vi "IcRn Curve Array.vi"() -> ()   [LabVIEW 2016]
panel:
  out "SC-fitting Clusters":cluster{"Rn":dbl, "Rc":dbl, "Rn/Rc ratio":dbl}[](array[cluster])=[{"Rn"=26609.67786588797, "Rc"=2146.640191844906, "Rn/Rc ratio"=12.39596554978251}, {"Rn"=26578.792114511656, "Rc"=2137.411881992016, "Rn/Rc ratio"=12.435035258501918}, {"Rn"=26563.358623435608, "Rc"=2083.2272039529967, "Rn/Rc ratio"=12.751061705142245}, {"Rn"=25938.706790932443, "Rc"=2244.184409808236, "Rn/Rc ratio"=11.558188657566197}, {"Rn"=25908.041740086435, "Rc"=2057.919835889771, "Rn/Rc ratio"=12.589431953691589}, {"Rn"=25865.50185276808, "Rc"=2204.392899899708, "Rn/Rc ratio"=11.733616930967646}, {"Rn"=25488.748575504553, "Rc"=2145.43014835337, "Rn/Rc ratio"=11.880484011594278}, {"Rn"=25365.459659139524, "Rc"=2113.116572134784, "Rn/Rc ratio"=12.003814646872025}, {"Rn"=25357.80891823078, "Rc"=2012.1993643655096, "Rn/Rc ratio"=12.602036044388997}, {"Rn"=24803.296836656464, "Rc"=1935.449110044589, "Rn/Rc ratio"=12.815266858700845}, {"Rn"=24789.427309484585, "Rc"=2110.7215877648796, "Rn/Rc ratio"=11.744527299659174}, {"Rn"=24753.340817673175, "Rc"=1907.8722974852653, "Rn/Rc ratio"=12.974317437440725}, {"Rn"=24193.381040172608, "Rc"=1986.2611655574085, "Rn/Rc ratio"=12.18036251208847}, {"Rn"=24141.67211311363, "Rc"=1914.2262988636805, "Rn/Rc ratio"=12.611712694285186}, {"Rn"=24054.376770789982, "Rc"=2034.7991063607624, "Rn/Rc ratio"=11.821499574870185}, {"Rn"=23498.377622554053, "Rc"=1747.9097873838214, "Rn/Rc ratio"=13.443701609866936}, {"Rn"=23433.481724089263, "Rc"=1853.1661496580136, "Rn/Rc ratio"=12.645105636326088}, {"Rn"=23378.696455272377, "Rc"=1802.771292074766, "Rn/Rc ratio"=12.968198771551547}, {"Rn"=22737.05296381861, "Rc"=1678.3245594247633, "Rn/Rc ratio"=13.547470801244552}, {"Rn"=22680.76965817146, "Rc"=1749.9212441766977, "Rn/Rc ratio"=12.961023093837746}, {"Rn"=22666.430402112397, "Rc"=1723.1362618386952, "Rn/Rc ratio"=13.154171787857267}, {"Rn"=22027.13711147753, "Rc"=1754.0754738398637, "Rn/Rc ratio"=12.557690612512646}, {"Rn"=21965.31458464643, "Rc"=1772.3528948958199, "Rn/Rc ratio"=12.393307590099072}, {"Rn"=21904.088799010322, "Rc"=1647.9899361875666, "Rn/Rc ratio"=13.2913971851569}, {"Rn"=21327.67605888909, "Rc"=1699.7562893724967, "Rn/Rc ratio"=12.547490597468348}, {"Rn"=21242.85250961181, "Rc"=1778.1623981981945, "Rn/Rc ratio"=11.946519919180112}, {"Rn"=21190.69234118089, "Rc"=1678.9409582743576, "Rn/Rc ratio"=12.621463689206214}, {"Rn"=20522.79001382321, "Rc"=1750.8462305265753, "Rn/Rc ratio"=11.721640459339987}, {"Rn"=20484.445522882474, "Rc"=1809.3684443337136, "Rn/Rc ratio"=11.321323518729606}, {"Rn"=20413.32456904895, "Rc"=1657.0773651102954, "Rn/Rc ratio"=12.318872370627206}, {"Rn"=19783.027782642876, "Rc"=1735.823288979653, "Rn/Rc ratio"=11.396913446340314}, {"Rn"=19715.891712150584, "Rc"=1800.9327427343387, "Rn/Rc ratio"=10.947600231986529}, {"Rn"=19681.22954295286, "Rc"=1875.9645987166225, "Rn/Rc ratio"=10.491258500516004}, {"Rn"=19073.25011455856, "Rc"=1794.1581209072158, "Rn/Rc ratio"=10.630752045931255}, {"Rn"=18990.747145177967, "Rc"=1751.6053469823771, "Rn/Rc ratio"=10.841909781729521}, {"Rn"=18936.08683536125, "Rc"=1762.5785362990346, "Rn/Rc ratio"=10.743400333878002}, {"Rn"=18450.3221338972, "Rc"=1708.93301365366, "Rn/Rc ratio"=10.796398680631038}, {"Rn"=18428.466285582617, "Rc"=1674.3218759950107, "Rn/Rc ratio"=11.006525417719342}, {"Rn"=18355.767337683894, "Rc"=1858.6237983654753, "Rn/Rc ratio"=9.875999303262155}, {"Rn"=17859.23397265431, "Rc"=1739.1190161552418, "Rn/Rc ratio"=10.269126958393349}, {"Rn"=17778.957863612708, "Rc"=1743.0073597486146, "Rn/Rc ratio"=10.200162244970027}, {"Rn"=17766.767929712023, "Rc"=1826.0747012887841, "Rn/Rc ratio"=9.729485829453097}, {"Rn"=17124.26563957245, "Rc"=1800.6179257907434, "Rn/Rc ratio"=9.51021612875053}, {"Rn"=17040.07209132531, "Rc"=1840.0009129073826, "Rn/Rc ratio"=9.260904150531273}, {"Rn"=16996.11181161611, "Rc"=1842.768006105162, "Rn/Rc ratio"=9.22314244403383}, {"Rn"=16503.730435302114, "Rc"=1885.2441857597194, "Rn/Rc ratio"=8.754160633388405}, {"Rn"=16378.924486528076, "Rc"=1866.7278065970531, "Rn/Rc ratio"=8.77413644809095}, {"Rn"=16336.813010769789, "Rc"=1877.4399266184203, "Rn/Rc ratio"=8.701643540837598}, {"Rn"=15797.875553425325, "Rc"=1812.5608870279023, "Rn/Rc ratio"=8.7157764831445}, {"Rn"=15734.825878147443, "Rc"=1872.8361883043326, "Rn/Rc ratio"=8.401602861163083}, {"Rn"=15694.731752981366, "Rc"=1910.4003923466507, "Rn/Rc ratio"=8.215414850131316}, {"Rn"=15300.779487653343, "Rc"=1885.4328596855091, "Rn/Rc ratio"=8.115260858562483}, {"Rn"=15231.177407861678, "Rc"=1936.904865101264, "Rn/Rc ratio"=7.863668310351098}, {"Rn"=15191.108179437479, "Rc"=1919.9426274461057, "Rn/Rc ratio"=7.912271940982208}, {"Rn"=14806.152885467243, "Rc"=1867.241081445293, "Rn/Rc ratio"=7.929427556299745}, {"Rn"=14756.205731190325, "Rc"=1834.3880543575835, "Rn/Rc ratio"=8.044211635666183}, {"Rn"=14732.965553995622, "Rc"=1901.6404450592686, "Rn/Rc ratio"=7.747503263444966}, {"Rn"=14331.684473181096, "Rc"=1980.624550270427, "Rn/Rc ratio"=7.23594205233107}, {"Rn"=14240.534552208328, "Rc"=1957.7503878737575, "Rn/Rc ratio"=7.273927585668601}, {"Rn"=14224.099719417836, "Rc"=1933.6717752448858, "Rn/Rc ratio"=7.356005244280124}, {"Rn"=13925.05115218171, "Rc"=1968.8315523994395, "Rn/Rc ratio"=7.072748877480695}, {"Rn"=13914.525766155477, "Rc"=1952.9090448194245, "Rn/Rc ratio"=7.125024999534519}, {"Rn"=13900.160543802975, "Rc"=1970.0644207332862, "Rn/Rc ratio"=7.055688330551717}, {"Rn"=13569.240810667905, "Rc"=2016.888834974567, "Rn/Rc ratio"=6.727807985926509}, {"Rn"=13555.992121061312, "Rc"=1964.544925126344, "Rn/Rc ratio"=6.900321773089256}, {"Rn"=13556.977493365734, "Rc"=2007.8894139072875, "Rn/Rc ratio"=6.751854658660855}, {"Rn"=13267.959781743146, "Rc"=2017.4672930967038, "Rn/Rc ratio"=6.576542691493918}, {"Rn"=13233.202853717605, "Rc"=2004.1695247062132, "Rn/Rc ratio"=6.60283608276971}, {"Rn"=13204.171960570418, "Rc"=2007.485522874923, "Rn/Rc ratio"=6.57746808637539}, {"Rn"=12929.525312561722, "Rc"=2011.982125208965, "Rn/Rc ratio"=6.426262515239223}, {"Rn"=12902.37901238455, "Rc"=2032.3267630250373, "Rn/Rc ratio"=6.348575065350158}, {"Rn"=12867.464844428734, "Rc"=2084.56046668184, "Rn/Rc ratio"=6.172747229017011}, {"Rn"=12635.505659805094, "Rc"=2052.0589191286263, "Rn/Rc ratio"=6.157477030518479}, {"Rn"=12578.747677887168, "Rc"=2023.2906359397762, "Rn/Rc ratio"=6.216975186090654}, {"Rn"=12564.870248569116, "Rc"=2027.8736517600116, "Rn/Rc ratio"=6.196081416445221}, {"Rn"=12287.456007341623, "Rc"=2093.781580679471, "Rn/Rc ratio"=5.868547187884858}, {"Rn"=12260.101827231643, "Rc"=2057.114850581173, "Rn/Rc ratio"=5.95985286080062}, {"Rn"=12239.950999851239, "Rc"=2059.2985694862946, "Rn/Rc ratio"=5.943747633887093}, {"Rn"=11968.212813789605, "Rc"=2113.6196057668526, "Rn/Rc ratio"=5.662425150266034}, {"Rn"=11901.353165405668, "Rc"=2068.2746198260493, "Rn/Rc ratio"=5.754242232304056}, {"Rn"=11872.797453714444, "Rc"=2091.1697936758906, "Rn/Rc ratio"=5.6775865305725635}, {"Rn"=11654.569767254134, "Rc"=2073.6782578342772, "Rn/Rc ratio"=5.6202401328285205}, {"Rn"=11583.170493913314, "Rc"=2137.4139727042425, "Rn/Rc ratio"=5.419245238328053}, {"Rn"=11565.794206204415, "Rc"=2090.415090416247, "Rn/Rc ratio"=5.532773973565898}, {"Rn"=11389.764008623597, "Rc"=2169.6812982806573, "Rn/Rc ratio"=5.24951015508559}, {"Rn"=11336.004809315062, "Rc"=2221.1633517014097, "Rn/Rc ratio"=5.103634003609725}, {"Rn"=11312.595295934347, "Rc"=2232.5217076006597, "Rn/Rc ratio"=5.067182664974954}, {"Rn"=11107.690306718008, "Rc"=2265.135879507835, "Rn/Rc ratio"=4.903763349124764}, {"Rn"=11098.45825051801, "Rc"=2293.6519573759015, "Rn/Rc ratio"=4.838771730308823}, {"Rn"=11042.554973244516, "Rc"=2261.662027967936, "Rn/Rc ratio"=4.882495632278913}, {"Rn"=10869.313335071296, "Rc"=2236.1809824862203, "Rn/Rc ratio"=4.860659052285932}, {"Rn"=10827.650137466882, "Rc"=2257.009387478776, "Rn/Rc ratio"=4.797343864644738}, {"Rn"=10767.742631637293, "Rc"=2256.68945035892, "Rn/Rc ratio"=4.771477364740955}, {"Rn"=10550.21488969895, "Rc"=2365.489605338067, "Rn/Rc ratio"=4.460055485296098}, {"Rn"=10477.3548184157, "Rc"=2334.973260367238, "Rn/Rc ratio"=4.487141243222569}, {"Rn"=10455.293240880203, "Rc"=2326.409930528063, "Rn/Rc ratio"=4.494174953296815}, {"Rn"=10280.682357607753, "Rc"=2395.365182096868, "Rn/Rc ratio"=4.29190606695226}, {"Rn"=10226.825214613966, "Rc"=2400.801791865318, "Rn/Rc ratio"=4.2597540743537055}, {"Rn"=10191.78568335829, "Rc"=2456.119197273396, "Rn/Rc ratio"=4.149548480656992}, {"Rn"=10006.21595421555, "Rc"=2472.905532503837, "Rn/Rc ratio"=4.046339750020364}, {"Rn"=9957.582001659894, "Rc"=2440.5490001667, "Rn/Rc ratio"=4.080058216810951}, {"Rn"=9917.824146352148, "Rc"=2422.710142005342, "Rn/Rc ratio"=4.0936899443294115}, {"Rn"=9748.514690463888, "Rc"=2518.231072664875, "Rn/Rc ratio"=3.871175602701022}, {"Rn"=9698.854169291048, "Rc"=2580.2945829373466, "Rn/Rc ratio"=3.7588166224997845}, {"Rn"=9664.809079681876, "Rc"=2522.333293159518, "Rn/Rc ratio"=3.8316938946540136}, {"Rn"=9473.25246470378, "Rc"=2702.5208526799665, "Rn/Rc ratio"=3.5053392669697954}, {"Rn"=9426.934255914573, "Rc"=2717.4330794274415, "Rn/Rc ratio"=3.4690584755451686}, {"Rn"=9399.40513012256, "Rc"=2697.561766580609, "Rn/Rc ratio"=3.484407751685002}, {"Rn"=9243.88186880994, "Rc"=2715.792185019114, "Rn/Rc ratio"=3.403751553525028}, {"Rn"=9188.754086177987, "Rc"=2793.5147814219454, "Rn/Rc ratio"=3.2893164365147047}, {"Rn"=9172.363064116218, "Rc"=2723.3582417778516, "Rn/Rc ratio"=3.368033967550429}, {"Rn"=8968.91761481306, "Rc"=2791.9644234624852, "Rn/Rc ratio"=3.2124039760113265}, {"Rn"=8932.625457914024, "Rc"=2813.723774279795, "Rn/Rc ratio"=3.1746632485985344}, {"Rn"=8919.401104724888, "Rc"=2832.88027299338, "Rn/Rc ratio"=3.1485273803330025}, {"Rn"=8753.717365168128, "Rc"=2948.1760690172496, "Rn/Rc ratio"=2.9691976192202483}, {"Rn"=8700.555867162924, "Rc"=2893.133644499764, "Rn/Rc ratio"=3.0073121176769178}, {"Rn"=8661.395277758254, "Rc"=2943.390451031439, "Rn/Rc ratio"=2.9426592977914567}, {"Rn"=8492.711609421736, "Rc"=2955.4709490890928, "Rn/Rc ratio"=2.8735561119419155}, {"Rn"=8458.010714831798, "Rc"=3024.164142525516, "Rn/Rc ratio"=2.796809404587547}, {"Rn"=8431.276070124082, "Rc"=3001.717149287295, "Rn/Rc ratio"=2.8088176369735374}, {"Rn"=8309.163801318718, "Rc"=3088.8502750646994, "Rn/Rc ratio"=2.6900506859772197}, {"Rn"=8251.83370188871, "Rc"=3075.5139455401554, "Rn/Rc ratio"=2.6830747146683587}, {"Rn"=8243.932270179163, "Rc"=3124.563747340813, "Rn/Rc ratio"=2.638426653063242}, {"Rn"=8090.6157777360895, "Rc"=3159.0436097894453, "Rn/Rc ratio"=2.561096577668119}, {"Rn"=8051.922432176443, "Rc"=3150.5956848083456, "Rn/Rc ratio"=2.555682555842214}, {"Rn"=8023.273315432865, "Rc"=3063.6901827522306, "Rn/Rc ratio"=2.6188265904306456}, {"Rn"=7895.293592904535, "Rc"=3224.7362048629902, "Rn/Rc ratio"=2.4483533198772096}, {"Rn"=7871.932381268901, "Rc"=3193.328946850622, "Rn/Rc ratio"=2.4651179105843415}, {"Rn"=7820.928301257313, "Rc"=3182.9637678964223, "Rn/Rc ratio"=2.457121372269361}, {"Rn"=7707.334223336343, "Rc"=3251.4358180420054, "Rn/Rc ratio"=2.3704402161558433}, {"Rn"=7663.960681742132, "Rc"=3223.469952980636, "Rn/Rc ratio"=2.37754990539171}, {"Rn"=7647.647756011226, "Rc"=3216.7866659301435, "Rn/Rc ratio"=2.37741838369623}, {"Rn"=7503.215694197473, "Rc"=3268.767339431267, "Rn/Rc ratio"=2.2954266593666337}, {"Rn"=7493.358403764781, "Rc"=3255.2583719053846, "Rn/Rc ratio"=2.301924316802764}, {"Rn"=7462.350795879372, "Rc"=3263.0643410531193, "Rn/Rc ratio"=2.2869150025619716}, {"Rn"=7333.204228214964, "Rc"=3259.977007083517, "Rn/Rc ratio"=2.2494650153301206}, {"Rn"=7313.634323329306, "Rc"=3272.968304949994, "Rn/Rc ratio"=2.234557026497404}, {"Rn"=7309.533866404526, "Rc"=3254.2165118238777, "Rn/Rc ratio"=2.246173184803792}, {"Rn"=7171.939058896087, "Rc"=3355.665266873474, "Rn/Rc ratio"=2.1372629533988934}, {"Rn"=7168.6158228906515, "Rc"=3330.261606676283, "Rn/Rc ratio"=2.15256837736696}, {"Rn"=7144.294179640347, "Rc"=3348.3488758190606, "Rn/Rc ratio"=2.1336767596813626}, {"Rn"=7031.674152349298, "Rc"=3400.8306990079313, "Rn/Rc ratio"=2.0676342854704686}, {"Rn"=7029.473963915299, "Rc"=3328.0083795732694, "Rn/Rc ratio"=2.112216425613882}, {"Rn"=7007.750803691114, "Rc"=3381.8897922381184, "Rn/Rc ratio"=2.0721404996031576}, {"Rn"=6941.985992286857, "Rc"=3400.3290612853143, "Rn/Rc ratio"=2.0415629979243266}, {"Rn"=6937.266120864143, "Rc"=3376.285920303337, "Rn/Rc ratio"=2.054703388462099}, {"Rn"=6926.842840126617, "Rc"=3438.190738351181, "Rn/Rc ratio"=2.014676720189309}, {"Rn"=6827.952061576165, "Rc"=3401.9128691800297, "Rn/Rc ratio"=2.0070919874035225}, {"Rn"=6827.449574060449, "Rc"=3440.9651961524573, "Rn/Rc ratio"=1.9841669952647636}, {"Rn"=6827.205706471883, "Rc"=3448.1065352464957, "Rn/Rc ratio"=1.9799868816941366}, {"Rn"=6720.95595907641, "Rc"=3478.6657769583335, "Rn/Rc ratio"=1.9320499266109612}, {"Rn"=6716.634412018881, "Rc"=3515.681917820842, "Rn/Rc ratio"=1.9104784132980142}, {"Rn"=6699.265788078224, "Rc"=3502.6556882720974, "Rn/Rc ratio"=1.91262470088319}, {"Rn"=7550.842918113843, "Rc"=3113.6618501963203, "Rn/Rc ratio"=2.425068386163306}, {"Rn"=7376.500026274158, "Rc"=3190.400072867101, "Rn/Rc ratio"=2.3120924830111216}, {"Rn"=7238.065583726423, "Rc"=3291.099294689989, "Rn/Rc ratio"=2.1992850824661083}, {"Rn"=8069.912478127117, "Rc"=2830.7038853913714, "Rn/Rc ratio"=2.850850108262516}, {"Rn"=8010.45076832988, "Rc"=2835.140263739777, "Rn/Rc ratio"=2.825416037005328}, {"Rn"=7932.990096204382, "Rc"=2870.226757364067, "Rn/Rc ratio"=2.7638896738213847}, {"Rn"=8840.66446644865, "Rc"=2575.0527344264106, "Rn/Rc ratio"=3.4331974441750206}, {"Rn"=8816.657274861956, "Rc"=2583.470857334935, "Rn/Rc ratio"=3.4127179138986192}, {"Rn"=8769.266362570657, "Rc"=2615.7036408845183, "Rn/Rc ratio"=3.352545841013269}, {"Rn"=9725.385147433728, "Rc"=2366.3079205647205, "Rn/Rc ratio"=4.109940664490004}, {"Rn"=9714.746308846783, "Rc"=2339.050606925809, "Rn/Rc ratio"=4.153286072597966}, {"Rn"=9680.198808964842, "Rc"=2362.88212877652, "Rn/Rc ratio"=4.096776005486641}, {"Rn"=10675.26004842822, "Rc"=2219.324837390063, "Rn/Rc ratio"=4.810138591961318}, {"Rn"=10664.548179659814, "Rc"=2182.293091134107, "Rn/Rc ratio"=4.8868542099070655}, {"Rn"=10642.72977053403, "Rc"=2228.9540755262074, "Rn/Rc ratio"=4.774764041749722}, {"Rn"=11690.937863973895, "Rc"=2111.3142898151946, "Rn/Rc ratio"=5.537279750518438}, {"Rn"=11684.64710716953, "Rc"=2092.462938582589, "Rn/Rc ratio"=5.584159648287287}, {"Rn"=11681.044366211387, "Rc"=2180.421565855196, "Rn/Rc ratio"=5.357241255146866}, {"Rn"=12830.05033002019, "Rc"=1992.6611448488106, "Rn/Rc ratio"=6.438651329749116}, {"Rn"=12825.415717937522, "Rc"=2146.2786558309067, "Rn/Rc ratio"=5.975652640953237}, {"Rn"=12817.2928306027, "Rc"=2006.1549038193114, "Rn/Rc ratio"=6.388984622374463}, {"Rn"=14019.251097543482, "Rc"=2050.672150601363, "Rn/Rc ratio"=6.836417558717182}, {"Rn"=14016.944910803903, "Rc"=1915.9517496215685, "Rn/Rc ratio"=7.315917487782496}, {"Rn"=13989.922360015049, "Rc"=1881.637717437653, "Rn/Rc ratio"=7.434971264854334}, {"Rn"=15169.651926141038, "Rc"=1911.7675836551032, "Rn/Rc ratio"=7.934882909322179}, {"Rn"=15144.715419523729, "Rc"=1997.790205892835, "Rn/Rc ratio"=7.580733640024722}, {"Rn"=15150.761941819905, "Rc"=1958.5165848362258, "Rn/Rc ratio"=7.735835406819818}, {"Rn"=16328.761773666572, "Rc"=1773.6861628237248, "Rn/Rc ratio"=9.206116682824561}, {"Rn"=16365.450013743182, "Rc"=1792.540273233297, "Rn/Rc ratio"=9.12975304271629}, {"Rn"=16340.152301706192, "Rc"=1968.5824129726768, "Rn/Rc ratio"=8.30046646461277}, {"Rn"=17581.093499879516, "Rc"=1775.3612726157971, "Rn/Rc ratio"=9.902825847933324}, {"Rn"=17564.370302623367, "Rc"=1760.6583395772593, "Rn/Rc ratio"=9.97602425626805}, {"Rn"=17589.551803826154, "Rc"=1801.1883131263248, "Rn/Rc ratio"=9.765526278202387}, {"Rn"=18753.320180612016, "Rc"=1693.9410828170157, "Rn/Rc ratio"=11.070821984803235}, {"Rn"=18719.410939340483, "Rc"=1750.4870316409679, "Rn/Rc ratio"=10.69383011754863}, {"Rn"=18773.30048872475, "Rc"=1776.077800067042, "Rn/Rc ratio"=10.570089040027476}, {"Rn"=19867.387923801773, "Rc"=1703.5244805579002, "Rn/Rc ratio"=11.662519764491584}, {"Rn"=19847.062782574056, "Rc"=1734.977532887819, "Rn/Rc ratio"=11.439377401930505}, {"Rn"=19855.836409861076, "Rc"=1815.3475119817938, "Rn/Rc ratio"=10.937760554828806}, {"Rn"=21020.249520976548, "Rc"=1621.8575575548239, "Rn/Rc ratio"=12.960601517107026}, {"Rn"=21032.885158751124, "Rc"=1646.333026368005, "Rn/Rc ratio"=12.775595715984647}, {"Rn"=20969.400889922497, "Rc"=1705.7025019941427, "Rn/Rc ratio"=12.293703541741364}, {"Rn"=22058.101382596084, "Rc"=1735.6814427739314, "Rn/Rc ratio"=12.708611637480704}, {"Rn"=21999.99443827097, "Rc"=1524.611849856769, "Rn/Rc ratio"=14.429898626550607}, {"Rn"=22103.063968275237, "Rc"=1681.9791202830133, "Rn/Rc ratio"=13.141104845912789}, {"Rn"=23150.48343465833, "Rc"=1600.7270370407525, "Rn/Rc ratio"=14.462480422306347}, {"Rn"=23171.75613824951, "Rc"=1631.0603075348222, "Rn/Rc ratio"=14.206560009587388}, {"Rn"=23122.809819249895, "Rc"=1737.891124042916, "Rn/Rc ratio"=13.305096907025167}, {"Rn"=24307.833027880424, "Rc"=1666.941071536739, "Rn/Rc ratio"=14.582298944419936}, {"Rn"=24305.998925916287, "Rc"=1606.849177207543, "Rn/Rc ratio"=15.126496793032173}, {"Rn"=24337.277550520284, "Rc"=1618.623552901965, "Rn/Rc ratio"=15.035786120180298}, {"Rn"=25405.283882227224, "Rc"=1569.717154610774, "Rn/Rc ratio"=16.184625241307693}, {"Rn"=25339.14434654796, "Rc"=1678.2220425439139, "Rn/Rc ratio"=15.09880320016409}, {"Rn"=25501.83951005843, "Rc"=1578.6742163015424, "Rn/Rc ratio"=16.153959598962203}, {"Rn"=26562.128547128887, "Rc"=1512.5673225425685, "Rn/Rc ratio"=17.560956230681324}, {"Rn"=26619.041980553437, "Rc"=1652.5419505810505, "Rn/Rc ratio"=16.10793721224076}, {"Rn"=26621.793547838293, "Rc"=1584.443285042716, "Rn/Rc ratio"=16.801985782104268}, {"Rn"=27822.73766879678, "Rc"=1555.1770627746844, "Rn/Rc ratio"=17.890398678563695}, {"Rn"=27899.864254786327, "Rc"=1522.5955344816273, "Rn/Rc ratio"=18.323884198363242}, {"Rn"=27863.023544867498, "Rc"=1500.0979790907222, "Rn/Rc ratio"=18.574135778621972}, {"Rn"=28935.58003445011, "Rc"=1480.6830831536345, "Rn/Rc ratio"=19.54204810175965}, {"Rn"=29119.86647846061, "Rc"=1417.109207381416, "Rn/Rc ratio"=20.54878080445848}, {"Rn"=29058.267402154204, "Rc"=1528.53219415966, "Rn/Rc ratio"=19.0105694294058}, {"Rn"=30242.00830489417, "Rc"=1606.8294191455718, "Rn/Rc ratio"=18.820920220004}, {"Rn"=30332.949838943012, "Rc"=1645.6371230805794, "Rn/Rc ratio"=18.43234417449256}, {"Rn"=30303.770516491975, "Rc"=1625.6783514323154, "Rn/Rc ratio"=18.640692662107867}, {"Rn"=31463.448172240427, "Rc"=1457.2602316184577, "Rn/Rc ratio"=21.590823306347}, {"Rn"=31570.513722895146, "Rc"=1387.0450979211305, "Rn/Rc ratio"=22.76098576045744}, {"Rn"=31589.166855000723, "Rc"=1414.4141350562893, "Rn/Rc ratio"=22.33374658246297}, {"Rn"=32818.666395995526, "Rc"=1539.1335280866954, "Rn/Rc ratio"=21.322819493635862}, {"Rn"=32880.60138763699, "Rc"=1562.1757547226453, "Rn/Rc ratio"=21.04795269561378}, {"Rn"=32760.475448269164, "Rc"=1539.8691448296977, "Rn/Rc ratio"=21.274843747773335}, {"Rn"=34089.18302702669, "Rc"=1419.5274299035673, "Rn/Rc ratio"=24.014458832502072}, {"Rn"=34033.94748928295, "Rc"=1523.7820110544121, "Rn/Rc ratio"=22.335181307024662}, {"Rn"=34081.636013545, "Rc"=1396.124671560047, "Rn/Rc ratio"=24.411599270330033}, {"Rn"=35339.79090900418, "Rc"=1302.7160898022455, "Rn/Rc ratio"=27.127776486102064}, {"Rn"=35356.20590883877, "Rc"=1336.4629400940091, "Rn/Rc ratio"=26.455058983043518}, {"Rn"=35382.48760468083, "Rc"=1389.706377769346, "Rn/Rc ratio"=25.460405284657455}, {"Rn"=36446.758146736895, "Rc"=1317.173751847343, "Rn/Rc ratio"=27.67042548154344}, {"Rn"=36661.25917846269, "Rc"=1486.9221846055668, "Rn/Rc ratio"=24.655802138151405}, {"Rn"=36547.713589699735, "Rc"=1429.206935965438, "Rn/Rc ratio"=25.572023665706276}, {"Rn"=37889.8719978444, "Rc"=1192.123990847668, "Rn/Rc ratio"=31.783499274184177}, {"Rn"=37885.6272839512, "Rc"=1179.1398893362887, "Rn/Rc ratio"=32.129883507949316}, {"Rn"=38021.67622185228, "Rc"=1307.176759287812, "Rn/Rc ratio"=29.086866754399455}, {"Rn"=39112.909925950706, "Rc"=1127.251997228521, "Rn/Rc ratio"=34.697574297596546}, {"Rn"=39139.051826896706, "Rc"=1110.7863282890992, "Rn/Rc ratio"=35.235446125071654}, {"Rn"=39235.900516596754, "Rc"=1411.7960948394114, "Rn/Rc ratio"=27.79147828784705}, {"Rn"=40400.155649211745, "Rc"=1325.9310839265488, "Rn/Rc ratio"=30.469272603197943}, {"Rn"=40380.75249187182, "Rc"=1391.8978602889642, "Rn/Rc ratio"=29.011290011961506}, {"Rn"=40499.658931168444, "Rc"=1290.6762207258196, "Rn/Rc ratio"=31.378635695630322}, {"Rn"=41694.5686923445, "Rc"=1271.9932102532262, "Rn/Rc ratio"=32.77892394098866}, {"Rn"=41721.64806182282, "Rc"=1517.5306342408544, "Rn/Rc ratio"=27.493117516335413}, {"Rn"=41701.022231542054, "Rc"=1270.030074002291, "Rn/Rc ratio"=32.834673040558904}, {"Rn"=42782.01332875257, "Rc"=1174.1183459694282, "Rn/Rc ratio"=36.437564812454205}, {"Rn"=42931.454419036345, "Rc"=1430.862453206742, "Rn/Rc ratio"=30.00390032097186}, {"Rn"=42951.82916326564, "Rc"=1257.0549303762505, "Rn/Rc ratio"=34.16861755628267}, {"Rn"=44239.35237071298, "Rc"=1401.4398328900888, "Rn/Rc ratio"=31.56707218709585}, {"Rn"=44327.62215382431, "Rc"=1517.0481689086425, "Rn/Rc ratio"=29.2196537079725}, {"Rn"=44268.0729307259, "Rc"=1299.203834938817, "Rn/Rc ratio"=34.07323142084984}, {"Rn"=45312.53497082396, "Rc"=1585.3800731362012, "Rn/Rc ratio"=28.581496474335417}, {"Rn"=45269.961721247644, "Rc"=1231.1273002317273, "Rn/Rc ratio"=36.7711460161161}, {"Rn"=45381.90420100819, "Rc"=1378.0852748063107, "Rn/Rc ratio"=32.93112917659366}, {"Rn"=46677.91873660844, "Rc"=1442.8367238446183, "Rn/Rc ratio"=32.35149061927763}, {"Rn"=46635.40741978568, "Rc"=1545.1084779114456, "Rn/Rc ratio"=30.18261053283696}, {"Rn"=46803.126604838806, "Rc"=1514.1929333127973, "Rn/Rc ratio"=30.909618962784023}, {"Rn"=47730.0368968397, "Rc"=1644.474082634305, "Rn/Rc ratio"=29.024499322227275}, {"Rn"=47953.021124481165, "Rc"=1842.0622503971674, "Rn/Rc ratio"=26.032247886379523}, {"Rn"=47878.269288228985, "Rc"=1693.1415177274205, "Rn/Rc ratio"=28.277771696539855}, {"Rn"=49041.360700655394, "Rc"=1987.3475741020482, "Rn/Rc ratio"=24.676790984996153}, {"Rn"=49099.83663298128, "Rc"=2055.3685483103995, "Rn/Rc ratio"=23.88858031000982}, {"Rn"=49119.1249156674, "Rc"=1828.8796309430218, "Rn/Rc ratio"=26.857494656627676}, {"Rn"=50232.609055324574, "Rc"=2117.3881994707867, "Rn/Rc ratio"=23.723854259639094}, {"Rn"=50406.79748543203, "Rc"=1989.2529516023826, "Rn/Rc ratio"=25.339561489567405}, {"Rn"=50059.97804726815, "Rc"=1916.2374022372533, "Rn/Rc ratio"=26.124100275269612}, {"Rn"=51436.45018793038, "Rc"=1937.8818153722286, "Rn/Rc ratio"=26.542614611433596}, {"Rn"=51466.467880199714, "Rc"=1722.069419720639, "Rn/Rc ratio"=29.886407185924487}, {"Rn"=51292.73061325326, "Rc"=2156.7832312915016, "Rn/Rc ratio"=23.782051839553066}, {"Rn"=52520.5565200649, "Rc"=2406.766333276112, "Rn/Rc ratio"=21.822042212371088}, {"Rn"=52452.30962292491, "Rc"=2329.7278148859095, "Rn/Rc ratio"=22.514350941675815}, {"Rn"=52538.85936867625, "Rc"=2487.3213463379047, "Rn/Rc ratio"=21.122666536846744}, {"Rn"=53684.137369906806, "Rc"=2971.270426012666, "Rn/Rc ratio"=18.06773860094213}, {"Rn"=53775.48786839241, "Rc"=2455.66899951783, "Rn/Rc ratio"=21.898508259440185}, {"Rn"=53677.48630055636, "Rc"=2472.2405010997336, "Rn/Rc ratio"=21.712081116978244}, {"Rn"=54762.76617976642, "Rc"=3314.5557055357585, "Rn/Rc ratio"=16.521902494595327}, {"Rn"=54764.000753055356, "Rc"=2943.4730392625247, "Rn/Rc ratio"=18.60523266989945}, {"Rn"=55043.61270306726, "Rc"=3614.956123371274, "Rn/Rc ratio"=15.22663369195588}, {"Rn"=55959.170526710455, "Rc"=3766.552286516182, "Rn/Rc ratio"=14.856868103766343}, {"Rn"=56030.18655552174, "Rc"=3536.9986586456284, "Rn/Rc ratio"=15.841167035380376}, {"Rn"=55882.48980643997, "Rc"=3704.205855281124, "Rn/Rc ratio"=15.086226843135009}, {"Rn"=56995.4549786711, "Rc"=4030.861542276598, "Rn/Rc ratio"=14.13976996750936}, {"Rn"=57202.58476788434, "Rc"=4131.675807842351, "Rn/Rc ratio"=13.844887021219787}, {"Rn"=57115.33801223602, "Rc"=3870.232994210082, "Rn/Rc ratio"=14.757596790085065}, {"Rn"=58230.1610385508, "Rc"=4259.749770669129, "Rn/Rc ratio"=13.669854844408832}, {"Rn"=58204.71818785964, "Rc"=4883.316387454577, "Rn/Rc ratio"=11.919096280017765}, {"Rn"=58094.64020429482, "Rc"=4431.609567945053, "Rn/Rc ratio"=13.109151271923405}, {"Rn"=59286.08339023979, "Rc"=5598.250313627349, "Rn/Rc ratio"=10.590109421496333}, {"Rn"=59279.71288795376, "Rc"=4569.173392910254, "Rn/Rc ratio"=12.97383745163512}, {"Rn"=59035.57241342334, "Rc"=5692.848386781651, "Rn/Rc ratio"=10.37012904655942}, {"Rn"=60108.74131172781, "Rc"=6626.4405405049065, "Rn/Rc ratio"=9.071045147738968}, {"Rn"=60348.841931070165, "Rc"=6005.768561238122, "Rn/Rc ratio"=10.048479443674886}, {"Rn"=60175.07314949414, "Rc"=6568.707974818762, "Rn/Rc ratio"=9.160868983699103}, {"Rn"=61469.54174611423, "Rc"=8197.681918357055, "Rn/Rc ratio"=7.49840532461568}, {"Rn"=61242.99103651691, "Rc"=8100.523540474841, "Rn/Rc ratio"=7.5603744289504204}, {"Rn"=61064.40097547228, "Rc"=7429.723148000197, "Rn/Rc ratio"=8.218933567115286}, {"Rn"=62001.81460691528, "Rc"=9219.196521987986, "Rn/Rc ratio"=6.725294819243693}, {"Rn"=62301.99331481748, "Rc"=9759.796080933154, "Rn/Rc ratio"=6.383534327784916}, {"Rn"=62372.0370034292, "Rc"=8894.084748712998, "Rn/Rc ratio"=7.012754967559156}, {"Rn"=63455.30310589003, "Rc"=9190.729882774918, "Rn/Rc ratio"=6.90427244791697}, {"Rn"=63643.48700971763, "Rc"=9196.053183448696, "Rn/Rc ratio"=6.9207393367694845}, {"Rn"=63737.251021554315, "Rc"=8680.755327551271, "Rn/Rc ratio"=7.342362342509862}, {"Rn"=65041.98748333938, "Rc"=9567.06643826341, "Rn/Rc ratio"=6.798529925871994}, {"Rn"=64731.5085143094, "Rc"=10817.039995291483, "Rn/Rc ratio"=5.984216434670315}, {"Rn"=64784.739371338655, "Rc"=9981.108217384291, "Rn/Rc ratio"=6.490736094665501}, {"Rn"=65870.2916438197, "Rc"=9242.12791403145, "Rn/Rc ratio"=7.127178097569399}, {"Rn"=65962.88923577876, "Rc"=9309.89379148612, "Rn/Rc ratio"=7.0852461599617484}, {"Rn"=65878.70140314334, "Rc"=9611.99933509268, "Rn/Rc ratio"=6.853797956750288}, {"Rn"=66938.77585704504, "Rc"=9888.82185831674, "Rn/Rc ratio"=6.769135577131253}, {"Rn"=66801.77837426163, "Rc"=10393.839735047934, "Rn/Rc ratio"=6.427054878382109}, {"Rn"=66883.78507526271, "Rc"=8411.690868504778, "Rn/Rc ratio"=7.951289000133174}, {"Rn"=67978.99405710607, "Rc"=10429.030189476196, "Rn/Rc ratio"=6.518246933996108}, {"Rn"=67974.19871114676, "Rc"=10663.56683353572, "Rn/Rc ratio"=6.374433599213308}, {"Rn"=68155.63063820021, "Rc"=9381.949349254397, "Rn/Rc ratio"=7.264548986679051}, {"Rn"=68792.33506188946, "Rc"=10723.92850330378, "Rn/Rc ratio"=6.4148446197395135}, {"Rn"=68575.00788832064, "Rc"=9740.404622619897, "Rn/Rc ratio"=7.040262755519481}, {"Rn"=68819.16828646393, "Rc"=10094.519835942907, "Rn/Rc ratio"=6.817478137139713}, {"Rn"=69555.92297661296, "Rc"=12473.244598500409, "Rn/Rc ratio"=5.576409764703508}, {"Rn"=69922.5112731253, "Rc"=12820.412855774855, "Rn/Rc ratio"=5.453998405490448}, {"Rn"=69685.66195665978, "Rc"=11275.650961101548, "Rn/Rc ratio"=6.180189702311608}, {"Rn"=70598.08128560062, "Rc"=11889.12448675304, "Rn/Rc ratio"=5.938038697825192}, {"Rn"=70790.81052417279, "Rc"=12954.244865839662, "Rn/Rc ratio"=5.464680593683089}, {"Rn"=70454.89668346469, "Rc"=11301.862191081762, "Rn/Rc ratio"=6.233919286244727}, {"Rn"=71261.1741093021, "Rc"=12411.091720893255, "Rn/Rc ratio"=5.741732936300729}, {"Rn"=71694.03934237703, "Rc"=13429.851481681308, "Rn/Rc ratio"=5.3384089496573885}, {"Rn"=71661.59154092136, "Rc"=12611.822963974239, "Rn/Rc ratio"=5.682096216036587}, {"Rn"=72544.93987732257, "Rc"=13984.455300778896, "Rn/Rc ratio"=5.187541331930319}, {"Rn"=72819.02138737592, "Rc"=15129.578513246037, "Rn/Rc ratio"=4.813023794656436}, {"Rn"=72605.46673016463, "Rc"=15476.144800174092, "Rn/Rc ratio"=4.6914440041519825}, {"Rn"=73765.98959006283, "Rc"=17002.62232952367, "Rn/Rc ratio"=4.338506623297407}, {"Rn"=73716.61624428055, "Rc"=15109.861916430607, "Rn/Rc ratio"=4.8787087964133145}, {"Rn"=73274.70810973497, "Rc"=17177.693904631098, "Rn/Rc ratio"=4.265689475930186}, {"Rn"=74738.46979926244, "Rc"=15097.692934928658, "Rn/Rc ratio"=4.950323875401802}, {"Rn"=74466.39156480864, "Rc"=18514.2600351432, "Rn/Rc ratio"=4.0221100612964715}, {"Rn"=74979.3527684867, "Rc"=16849.882703089963, "Rn/Rc ratio"=4.449844197119357}, {"Rn"=75936.88307936872, "Rc"=16294.748135077662, "Rn/Rc ratio"=4.660206003178386}, {"Rn"=75925.85772855344, "Rc"=18176.154823218432, "Rn/Rc ratio"=4.177223316317974}, {"Rn"=76005.38360260286, "Rc"=15907.565347459822, "Rn/Rc ratio"=4.777939423315943}, {"Rn"=77064.93250675398, "Rc"=19419.869860862338, "Rn/Rc ratio"=3.968354734552887}, {"Rn"=77342.24610505719, "Rc"=18069.02145192603, "Rn/Rc ratio"=4.280378232481043}, {"Rn"=77252.57233617116, "Rc"=21524.07572214045, "Rn/Rc ratio"=3.5891237948353036}, {"Rn"=78252.90679705876, "Rc"=23101.249250663954, "Rn/Rc ratio"=3.387388532453919}, {"Rn"=78662.322498667, "Rc"=21322.155615080475, "Rn/Rc ratio"=3.6892293592975967}, {"Rn"=78086.13842955435, "Rc"=21678.294620823857, "Rn/Rc ratio"=3.6020424943641984}, {"Rn"=79406.49623067894, "Rc"=21326.13368488862, "Rn/Rc ratio"=3.723436109140833}, {"Rn"=79324.1409368258, "Rc"=21745.20994039168, "Rn/Rc ratio"=3.6478903240884044}, {"Rn"=79409.94545871629, "Rc"=20283.461613766274, "Rn/Rc ratio"=3.9150095270139293}, {"Rn"=80252.11654711327, "Rc"=21781.508428986734, "Rn/Rc ratio"=3.6844150077463924}, {"Rn"=80499.13065510256, "Rc"=20257.975369011252, "Rn/Rc ratio"=3.9737006876927383}, {"Rn"=80493.18448261313, "Rc"=24132.451955192057, "Rn/Rc ratio"=3.335474763694501}, {"Rn"=80833.57209968234, "Rc"=26227.02656132668, "Rn/Rc ratio"=3.0820715383297124}, {"Rn"=80930.53738374737, "Rc"=25039.411870821066, "Rn/Rc ratio"=3.232126129849614}, {"Rn"=81462.88269933553, "Rc"=22668.98275929681, "Rn/Rc ratio"=3.593583512957884}, {"Rn"=82020.85579944043, "Rc"=20595.6349288411, "Rn/Rc ratio"=3.9824388071951358}, {"Rn"=82038.97739378078, "Rc"=22426.984873938218, "Rn/Rc ratio"=3.658047564348073}, {"Rn"=81834.0563757893, "Rc"=27296.19905785503, "Rn/Rc ratio"=2.998001890385537}, {"Rn"=82712.70238807966, "Rc"=25759.533551142744, "Rn/Rc ratio"=3.2109549741598626}, {"Rn"=83231.84818319579, "Rc"=26506.000937947723, "Rn/Rc ratio"=3.1401133795342036}, {"Rn"=83223.86994013686, "Rc"=28006.755033778394, "Rn/Rc ratio"=2.9715641758483695}, {"Rn"=84037.90275029757, "Rc"=31652.24531974979, "Rn/Rc ratio"=2.655037641132559}, {"Rn"=83808.42611394833, "Rc"=28302.278885652282, "Rn/Rc ratio"=2.961190031818768}, {"Rn"=84277.04845583954, "Rc"=30960.26247191449, "Rn/Rc ratio"=2.722103810724835}, {"Rn"=85097.2485172775, "Rc"=29587.006503781882, "Rn/Rc ratio"=2.8761695951363033}, {"Rn"=85124.75972215163, "Rc"=28809.790712131195, "Rn/Rc ratio"=2.9547163522540756}, {"Rn"=85390.24733065226, "Rc"=28415.126070599574, "Rn/Rc ratio"=3.005098309910489}, {"Rn"=85797.11614641946, "Rc"=30694.099305615233, "Rn/Rc ratio"=2.7952315945861157}, {"Rn"=86366.72544395947, "Rc"=30396.32144490808, "Rn/Rc ratio"=2.8413545237865425}, {"Rn"=86079.10491245994, "Rc"=31417.654839855364, "Rn/Rc ratio"=2.7398322806469606}, {"Rn"=87062.45092372524, "Rc"=29284.913601684246, "Rn/Rc ratio"=2.9729454594914038}, {"Rn"=87381.34492839195, "Rc"=31138.38220626684, "Rn/Rc ratio"=2.806226230687276}, {"Rn"=87057.3860941763, "Rc"=29783.92320019177, "Rn/Rc ratio"=2.9229657056601517}, {"Rn"=88124.65861655651, "Rc"=31039.654075433344, "Rn/Rc ratio"=2.839099250345824}, {"Rn"=87982.55582677905, "Rc"=28271.509834118686, "Rn/Rc ratio"=3.1120572032767684}, {"Rn"=88221.54744800628, "Rc"=28698.99493862682, "Rn/Rc ratio"=3.0740291650167273}, {"Rn"=89204.57761998638, "Rc"=28784.243244427555, "Rn/Rc ratio"=3.0990767018777126}, {"Rn"=89002.79520432782, "Rc"=27473.081352426394, "Rn/Rc ratio"=3.2396364303877836}, {"Rn"=88939.9894010748, "Rc"=33142.93422434724, "Rn/Rc ratio"=2.6835279217896857}, {"Rn"=89822.33128380564, "Rc"=32518.694078390414, "Rn/Rc ratio"=2.7621752296472173}, {"Rn"=90388.92130011319, "Rc"=35087.821747083195, "Rn/Rc ratio"=2.5760767354453145}, {"Rn"=90196.26949082303, "Rc"=28773.422727904388, "Rn/Rc ratio"=3.1347076899318944}, {"Rn"=91036.34653256538, "Rc"=36364.41399670173, "Rn/Rc ratio"=2.5034459936800415}, {"Rn"=91307.05738085724, "Rc"=33012.40657653905, "Rn/Rc ratio"=2.765840689898279}, {"Rn"=91562.8219764573, "Rc"=37862.1567020132, "Rn/Rc ratio"=2.418320295303958}, {"Rn"=92882.00179338467, "Rc"=36944.60589549061, "Rn/Rc ratio"=2.5140883098369082}, {"Rn"=91976.14395879339, "Rc"=39357.115732695594, "Rn/Rc ratio"=2.336963526074269}, {"Rn"=92685.22304037827, "Rc"=35799.7793522289, "Rn/Rc ratio"=2.5889886674569036}, {"Rn"=93336.31835733357, "Rc"=36722.45865350133, "Rn/Rc ratio"=2.5416685532419914}, {"Rn"=93742.20865293522, "Rc"=37552.290615982165, "Rn/Rc ratio"=2.4963113332170144}, {"Rn"=93868.1989661781, "Rc"=39065.17019215576, "Rn/Rc ratio"=2.402861641315125}, {"Rn"=95067.45371532663, "Rc"=43754.910153380304, "Rn/Rc ratio"=2.1727265210252558}, {"Rn"=94664.61525823842, "Rc"=37298.71296463221, "Rn/Rc ratio"=2.5380129161025566}, {"Rn"=95364.90988545949, "Rc"=43332.294801578, "Rn/Rc ratio"=2.200781433850733}, {"Rn"=96270.92091320675, "Rc"=40183.73831038324, "Rn/Rc ratio"=2.395768162971809}, {"Rn"=96011.9834728037, "Rc"=39053.0675290334, "Rn/Rc ratio"=2.4585004340933034}, {"Rn"=96476.1034315838, "Rc"=38800.13039175614, "Rn/Rc ratio"=2.4864891549973263}, {"Rn"=97969.56261800119, "Rc"=45225.15794059015, "Rn/Rc ratio"=2.166262476002815}, {"Rn"=97858.65742735188, "Rc"=39910.296793651134, "Rn/Rc ratio"=2.451965164110708}, {"Rn"=98065.76956034846, "Rc"=44400.317119885236, "Rn/Rc ratio"=2.2086727285204115}, {"Rn"=99285.12271967578, "Rc"=43380.91692329334, "Rn/Rc ratio"=2.288681977267399}, {"Rn"=98672.09986367568, "Rc"=45115.32396809535, "Rn/Rc ratio"=2.1871083078879057}, {"Rn"=99697.57502511785, "Rc"=45788.97209480059, "Rn/Rc ratio"=2.1773272136073714}, {"Rn"=100135.6959057588, "Rc"=49044.58559959308, "Rn/Rc ratio"=2.041727841749561}, {"Rn"=100560.59786145971, "Rc"=50100.22814881069, "Rn/Rc ratio"=2.007188421632904}, {"Rn"=100273.27689740434, "Rc"=47084.18192112502, "Rn/Rc ratio"=2.1296595333307735}, {"Rn"=101365.81716040843, "Rc"=50877.41714587194, "Rn/Rc ratio"=1.992353834900461}, {"Rn"=101810.22989072799, "Rc"=48316.96000973403, "Rn/Rc ratio"=2.1071323582902797}, {"Rn"=101653.88158680875, "Rc"=50656.596670387895, "Rn/Rc ratio"=2.0067254468011293}, {"Rn"=103131.52901062828, "Rc"=55598.27839099307, "Rn/Rc ratio"=1.8549410520476763}, {"Rn"=102924.42093146371, "Rc"=55389.60018285015, "Rn/Rc ratio"=1.8581903568845655}, {"Rn"=102914.35402584617, "Rc"=49584.85344769911, "Rn/Rc ratio"=2.0755199797937833}, {"Rn"=105211.51352916924, "Rc"=59426.18282504677, "Rn/Rc ratio"=1.7704572046788944}, {"Rn"=104320.41576688085, "Rc"=51568.060330559885, "Rn/Rc ratio"=2.0229656709631803}, {"Rn"=104126.47467621695, "Rc"=57245.3194053915, "Rn/Rc ratio"=1.8189517633542993}, {"Rn"=105007.4597966593, "Rc"=58532.68455564625, "Rn/Rc ratio"=1.79399698807305}, {"Rn"=106110.03546280273, "Rc"=55888.236595931055, "Rn/Rc ratio"=1.8986112628668637}, {"Rn"=106202.31934844087, "Rc"=58886.11711722909, "Rn/Rc ratio"=1.8035204993566785}, {"Rn"=106767.00811660911, "Rc"=58133.545678304814, "Rn/Rc ratio"=1.8365817338482777}, {"Rn"=106753.7806085116, "Rc"=61272.26517990539, "Rn/Rc ratio"=1.7422855233940682}, {"Rn"=107290.73920473912, "Rc"=58951.805344545246, "Rn/Rc ratio"=1.8199737663278641}, {"Rn"=108454.70457393774, "Rc"=53765.70710061794, "Rn/Rc ratio"=2.017172477076773}, {"Rn"=108550.53188691405, "Rc"=60419.075307629064, "Rn/Rc ratio"=1.79662683240714}, {"Rn"=108824.70246959796, "Rc"=59192.64569650051, "Rn/Rc ratio"=1.8384835005952727}, {"Rn"=109457.77050686299, "Rc"=61378.597289303914, "Rn/Rc ratio"=1.783321472645279}, {"Rn"=109510.28368600634, "Rc"=60928.3935230257, "Rn/Rc ratio"=1.797360431711052}, {"Rn"=110273.82235425165, "Rc"=66221.62461170842, "Rn/Rc ratio"=1.6652237543377109}, {"Rn"=110829.87538445793, "Rc"=61606.46990661966, "Rn/Rc ratio"=1.7989973383063322}, {"Rn"=111489.38876753394, "Rc"=70906.05359558089, "Rn/Rc ratio"=1.5723536019001112}, {"Rn"=111602.65666424322, "Rc"=64837.28821294229, "Rn/Rc ratio"=1.7212727388861708}, {"Rn"=112325.42547476148, "Rc"=73321.80822592253, "Rn/Rc ratio"=1.5319511096706617}, {"Rn"=112891.80481569027, "Rc"=75170.10706966936, "Rn/Rc ratio"=1.5018177998743514}, {"Rn"=112712.76368344166, "Rc"=63920.02556517956, "Rn/Rc ratio"=1.763340403681596}, {"Rn"=114161.81155271968, "Rc"=69603.46381617292, "Rn/Rc ratio"=1.6401742857830772}, {"Rn"=114860.45752812564, "Rc"=68952.19760629936, "Rn/Rc ratio"=1.6657983576383093}, {"Rn"=114476.89800887888, "Rc"=63839.21404295858, "Rn/Rc ratio"=1.7932065694268302}, {"Rn"=115389.95632354294, "Rc"=75164.32464909712, "Rn/Rc ratio"=1.535169202440629}, {"Rn"=115606.71349615869, "Rc"=72862.39747059833, "Rn/Rc ratio"=1.5866443804955592}, {"Rn"=115837.02956942853, "Rc"=74811.68867654065, "Rn/Rc ratio"=1.5483814310122979}, {"Rn"=115908.2796691345, "Rc"=70218.72674239964, "Rn/Rc ratio"=1.6506747565268296}, {"Rn"=116888.83437799172, "Rc"=69109.29883056368, "Rn/Rc ratio"=1.6913618913218877}, {"Rn"=117415.3477825604, "Rc"=73254.4848719818, "Rn/Rc ratio"=1.602841764401911}, {"Rn"=118309.4392415309, "Rc"=78350.54039028574, "Rn/Rc ratio"=1.5100015730867817}, {"Rn"=118940.06218617066, "Rc"=80659.6655018344, "Rn/Rc ratio"=1.4745915625383503}, {"Rn"=118211.39604708832, "Rc"=84742.31905556394, "Rn/Rc ratio"=1.394951157397278}, {"Rn"=120544.35950944432, "Rc"=77173.05213069804, "Rn/Rc ratio"=1.562000674863732}, {"Rn"=120744.18916741264, "Rc"=76766.05621031742, "Rn/Rc ratio"=1.5728851412739961}, {"Rn"=121199.04631178576, "Rc"=86271.54643439276, "Rn/Rc ratio"=1.4048553818836949}, {"Rn"=121593.78901922598, "Rc"=83280.49305723248, "Rn/Rc ratio"=1.4600512623726138}, {"Rn"=123098.26842718446, "Rc"=84251.90573163336, "Rn/Rc ratio"=1.461073994210742}, {"Rn"=122659.60643259337, "Rc"=87525.0486213098, "Rn/Rc ratio"=1.4014228882442383}, {"Rn"=122096.18595525682, "Rc"=82431.9673347061, "Rn/Rc ratio"=1.4811752030556111}, {"Rn"=124711.82907691061, "Rc"=81556.25604593845, "Rn/Rc ratio"=1.5291509826868925}, {"Rn"=124318.81108257867, "Rc"=82952.5670878398, "Rn/Rc ratio"=1.4986734642091968}, {"Rn"=120387.38824054475, "Rc"=78182.64411091183, "Rn/Rc ratio"=1.5398224197912804}, {"Rn"=120561.28124501812, "Rc"=80452.8457051316, "Rn/Rc ratio"=1.4985334600455062}, {"Rn"=120680.53655015228, "Rc"=82530.69604596662, "Rn/Rc ratio"=1.462250318147536}, {"Rn"=118829.99702014572, "Rc"=77761.9324519052, "Rn/Rc ratio"=1.5281255657276858}, {"Rn"=117895.38438730301, "Rc"=84629.4710667216, "Rn/Rc ratio"=1.393077173959349}, {"Rn"=118295.56742802303, "Rc"=87255.2883504929, "Rn/Rc ratio"=1.3557409489364753}, {"Rn"=116194.10691382702, "Rc"=75666.90784721635, "Rn/Rc ratio"=1.5356000426030572}, {"Rn"=115920.06199149112, "Rc"=81877.4347730951, "Rn/Rc ratio"=1.4157754491544283}, {"Rn"=116255.5195064721, "Rc"=84665.77214752523, "Rn/Rc ratio"=1.373111194260457}, {"Rn"=114807.08981075096, "Rc"=71020.9593974507, "Rn/Rc ratio"=1.6165240625413455}, {"Rn"=114958.89014289742, "Rc"=70420.810035554, "Rn/Rc ratio"=1.6324562311177204}, {"Rn"=114921.0306928925, "Rc"=79047.62757920958, "Rn/Rc ratio"=1.4538201108911968}, {"Rn"=111366.4151577422, "Rc"=65108.782425067235, "Rn/Rc ratio"=1.7104668680590398}, {"Rn"=111261.04980685457, "Rc"=72094.34546191007, "Rn/Rc ratio"=1.5432701288014}, {"Rn"=112099.33651112558, "Rc"=69586.6768192498, "Rn/Rc ratio"=1.6109310235104586}, {"Rn"=109326.84075498083, "Rc"=60112.655093384485, "Rn/Rc ratio"=1.8186992503515698}, {"Rn"=108969.90071299585, "Rc"=57032.79361753022, "Rn/Rc ratio"=1.9106533943219235}, {"Rn"=108674.33461846146, "Rc"=62734.58303627706, "Rn/Rc ratio"=1.7322875096757904}, {"Rn"=106529.35695691765, "Rc"=61891.36870774524, "Rn/Rc ratio"=1.7212312343576641}, {"Rn"=106122.05693573147, "Rc"=60149.81403010234, "Rn/Rc ratio"=1.7642956781648909}, {"Rn"=106951.08322496775, "Rc"=60260.36229007496, "Rn/Rc ratio"=1.7748164657580041}, {"Rn"=103846.81592602677, "Rc"=54614.74565861863, "Rn/Rc ratio"=1.9014428186692276}, {"Rn"=103014.78436899843, "Rc"=60037.49587583426, "Rn/Rc ratio"=1.715840790262923}, {"Rn"=103396.88467017724, "Rc"=59596.545489249555, "Rn/Rc ratio"=1.7349476185465935}, {"Rn"=101038.63519096088, "Rc"=56695.75699910572, "Rn/Rc ratio"=1.7821198717313995}, {"Rn"=101274.27657156212, "Rc"=53436.93545031477, "Rn/Rc ratio"=1.8952111628056614}, {"Rn"=100382.52953055516, "Rc"=52178.72349022325, "Rn/Rc ratio"=1.9238211059219161}, {"Rn"=97834.25024030387, "Rc"=47030.6380983492, "Rn/Rc ratio"=2.0802237476709444}, {"Rn"=97798.95020878923, "Rc"=46118.1018579285, "Rn/Rc ratio"=2.1206195890296793}, {"Rn"=98799.25778309035, "Rc"=42437.87208651596, "Rn/Rc ratio"=2.328091700301873}, {"Rn"=96118.1213704926, "Rc"=39202.43853500901, "Rn/Rc ratio"=2.451840369181527}, {"Rn"=95467.79606350213, "Rc"=37639.82184608517, "Rn/Rc ratio"=2.5363509012843934}, {"Rn"=95547.60389569186, "Rc"=41368.79083144451, "Rn/Rc ratio"=2.3096542580854433}, {"Rn"=92681.72348917203, "Rc"=36281.04729422286, "Rn/Rc ratio"=2.5545492867823034}, {"Rn"=92076.99287029411, "Rc"=37675.06229854063, "Rn/Rc ratio"=2.4439771894912243}, {"Rn"=91909.30039690436, "Rc"=35027.72161936356, "Rn/Rc ratio"=2.6239017597449523}, {"Rn"=89797.21945940827, "Rc"=40667.360090176524, "Rn/Rc ratio"=2.2080906963296933}, {"Rn"=89834.65554301618, "Rc"=35597.60875031238, "Rn/Rc ratio"=2.523614891470143}, {"Rn"=89861.84560867204, "Rc"=34538.741891291415, "Rn/Rc ratio"=2.6017695112203776}, {"Rn"=88072.7311722756, "Rc"=30415.18420558886, "Rn/Rc ratio"=2.8956829778493347}, {"Rn"=87443.22370548677, "Rc"=32877.68713642051, "Rn/Rc ratio"=2.659652527948685}, {"Rn"=87078.01963976369, "Rc"=33696.641392822276, "Rn/Rc ratio"=2.5841750406113824}, {"Rn"=84980.41638572102, "Rc"=29049.309728572152, "Rn/Rc ratio"=2.9253850497568443}, {"Rn"=84886.16351956123, "Rc"=30116.37773679151, "Rn/Rc ratio"=2.8186046894962575}, {"Rn"=84994.58400539513, "Rc"=30844.848941074935, "Rn/Rc ratio"=2.7555519616181683}, {"Rn"=82492.5743051752, "Rc"=27423.353439543404, "Rn/Rc ratio"=3.0081140326997406}, {"Rn"=82266.30497695156, "Rc"=26253.875015224385, "Rn/Rc ratio"=3.133491910403553}, {"Rn"=82021.72251303925, "Rc"=26592.731497956025, "Rn/Rc ratio"=3.084366211847911}, {"Rn"=79574.18118377356, "Rc"=21298.58519080213, "Rn/Rc ratio"=3.7361252154034137}, {"Rn"=79199.78834026428, "Rc"=19812.20138593941, "Rn/Rc ratio"=3.9975259082754855}, {"Rn"=79167.08083302634, "Rc"=26582.74379669382, "Rn/Rc ratio"=2.978138052207861}, {"Rn"=77057.87987203925, "Rc"=23015.613889393357, "Rn/Rc ratio"=3.348069716600131}, {"Rn"=76811.2061053128, "Rc"=23402.81943263861, "Rn/Rc ratio"=3.282134715708163}, {"Rn"=76817.24396125166, "Rc"=21483.146512398864, "Rn/Rc ratio"=3.5756979973542085}, {"Rn"=74478.3425674592, "Rc"=13272.263074005547, "Rn/Rc ratio"=5.611578232903558}, {"Rn"=74336.07175959641, "Rc"=15642.210891979421, "Rn/Rc ratio"=4.752273976673745}, {"Rn"=74425.12923405303, "Rc"=13514.084144345274, "Rn/Rc ratio"=5.507227011398689}, {"Rn"=72885.56349919624, "Rc"=15681.668289021454, "Rn/Rc ratio"=4.647819489347478}, {"Rn"=72554.30093484622, "Rc"=14104.725789800768, "Rn/Rc ratio"=5.143971036098467}, {"Rn"=72534.24132268627, "Rc"=12952.031887060042, "Rn/Rc ratio"=5.600221027493987}, {"Rn"=70332.61738810502, "Rc"=9420.059486764616, "Rn/Rc ratio"=7.46626042934483}, {"Rn"=70388.58014530504, "Rc"=11475.93851619878, "Rn/Rc ratio"=6.13357940581056}, {"Rn"=70301.43783595796, "Rc"=12984.932190162635, "Rn/Rc ratio"=5.4140781643217375}, {"Rn"=68385.07968943534, "Rc"=10871.513420813912, "Rn/Rc ratio"=6.2902998913205215}, {"Rn"=68282.19849370589, "Rc"=13348.176755637302, "Rn/Rc ratio"=5.115470055853766}, {"Rn"=68341.1082766758, "Rc"=9776.56280675845, "Rn/Rc ratio"=6.990300131804218}, {"Rn"=66586.54028974638, "Rc"=8408.826604914839, "Rn/Rc ratio"=7.918648274995646}, {"Rn"=66321.15260997973, "Rc"=9670.290631201902, "Rn/Rc ratio"=6.858237786151914}, {"Rn"=66281.7494521658, "Rc"=9224.200082799933, "Rn/Rc ratio"=7.185636570889136}, {"Rn"=65086.8035918342, "Rc"=9215.193454941586, "Rn/Rc ratio"=7.062988304052569}, {"Rn"=64305.98527731722, "Rc"=8552.271782339143, "Rn/Rc ratio"=7.519169983595727}, {"Rn"=64076.74824462419, "Rc"=9028.081274216227, "Rn/Rc ratio"=7.097493509238154}, {"Rn"=62641.66052029832, "Rc"=8017.155089401256, "Rn/Rc ratio"=7.813452505504241}, {"Rn"=62170.13387331633, "Rc"=8981.928684945542, "Rn/Rc ratio"=6.921690881104259}, {"Rn"=61943.966466716345, "Rc"=11280.289753511204, "Rn/Rc ratio"=5.491345330684888}, {"Rn"=60584.07456649259, "Rc"=7808.070175611345, "Rn/Rc ratio"=7.759161124822891}, {"Rn"=60191.947892648976, "Rc"=5237.207074192626, "Rn/Rc ratio"=11.493138812336962}, {"Rn"=60424.13048827607, "Rc"=6423.2774421636395, "Rn/Rc ratio"=9.407055982299683}, {"Rn"=58909.61468399183, "Rc"=5370.9767408759135, "Rn/Rc ratio"=10.968138110831717}, {"Rn"=58734.030691392334, "Rc"=4162.131565270012, "Rn/Rc ratio"=14.111526694995776}, {"Rn"=58590.86028651807, "Rc"=4635.922954012585, "Rn/Rc ratio"=12.638445648844366}, {"Rn"=56475.34456775305, "Rc"=3588.8599599389468, "Rn/Rc ratio"=15.73629096653685}, {"Rn"=56718.27771864169, "Rc"=2906.3089951660318, "Rn/Rc ratio"=19.51557037224168}, {"Rn"=56772.643334723994, "Rc"=3750.930044297047, "Rn/Rc ratio"=15.135617743935724}, {"Rn"=54907.94634455451, "Rc"=3485.709256166045, "Rn/Rc ratio"=15.75230241805885}, {"Rn"=54926.088516759846, "Rc"=2404.959875504768, "Rn/Rc ratio"=22.83867147897077}, {"Rn"=54646.68489705923, "Rc"=2604.065629687686, "Rn/Rc ratio"=20.985141186174015}, {"Rn"=53451.94010731803, "Rc"=1804.334404304382, "Rn/Rc ratio"=29.62418716830107}, {"Rn"=53705.779406219845, "Rc"=1971.8399386446192, "Rn/Rc ratio"=27.236378751479954}, {"Rn"=53177.52099218016, "Rc"=2007.4073002161995, "Rn/Rc ratio"=26.490648403267684}, {"Rn"=51505.35228404874, "Rc"=1764.9579725878475, "Rn/Rc ratio"=29.182197584302624}, {"Rn"=51160.28679138743, "Rc"=1709.3375301368026, "Rn/Rc ratio"=29.92989148684575}, {"Rn"=51541.81928534415, "Rc"=1625.7067999141207, "Rn/Rc ratio"=31.70425275213642}, {"Rn"=49524.47260383255, "Rc"=1623.2283061149428, "Rn/Rc ratio"=30.509862609755196}, {"Rn"=49881.36067385041, "Rc"=1704.1543912293341, "Rn/Rc ratio"=29.27044693284348}, {"Rn"=49502.45661180137, "Rc"=1475.921800574295, "Rn/Rc ratio"=33.54002670909766}, {"Rn"=48060.43864487917, "Rc"=1718.6895788187235, "Rn/Rc ratio"=27.963420059782816}, {"Rn"=48114.902421312756, "Rc"=1592.8434261181699, "Rn/Rc ratio"=30.206925321323585}, {"Rn"=47908.28087460886, "Rc"=1440.6129235222484, "Rn/Rc ratio"=33.2554845874038}, {"Rn"=46524.46483011354, "Rc"=1780.0976741352908, "Rn/Rc ratio"=26.135905633781302}, {"Rn"=46396.704923895355, "Rc"=1468.6580704488654, "Rn/Rc ratio"=31.591223210801648}, {"Rn"=46504.23300496034, "Rc"=1869.676390811075, "Rn/Rc ratio"=24.87287812667227}, {"Rn"=44791.07557992173, "Rc"=1543.7973954079848, "Rn/Rc ratio"=29.013571154577985}, {"Rn"=44709.7205439938, "Rc"=1507.728138697745, "Rn/Rc ratio"=29.653701749315683}, {"Rn"=44886.41837391495, "Rc"=1480.9042132998006, "Rn/Rc ratio"=30.31014293213301}, {"Rn"=43180.846775145124, "Rc"=1445.9406595723315, "Rn/Rc ratio"=29.86349853936385}, {"Rn"=42898.998846583585, "Rc"=1332.1357527588902, "Rn/Rc ratio"=32.20317355625248}, {"Rn"=42677.4928632744, "Rc"=1486.1912287760808, "Rn/Rc ratio"=28.716017183347585}, {"Rn"=41717.2352869645, "Rc"=2188.6023792356696, "Rn/Rc ratio"=19.061130373774656}, {"Rn"=41451.384534138786, "Rc"=1710.450329152098, "Rn/Rc ratio"=24.234193666814637}, {"Rn"=41291.03066771489, "Rc"=1461.3661563744797, "Rn/Rc ratio"=28.255088902670558}, {"Rn"=40187.88817328939, "Rc"=1806.9181734404312, "Rn/Rc ratio"=22.241122350753905}, {"Rn"=39667.590383900446, "Rc"=1632.9256767793775, "Rn/Rc ratio"=24.29234284694262}, {"Rn"=39750.70912136748, "Rc"=1825.7366674645186, "Rn/Rc ratio"=21.772421965195587}, {"Rn"=37946.722191298766, "Rc"=1904.8541422911671, "Rn/Rc ratio"=19.921064478803757}, {"Rn"=38037.472014065395, "Rc"=1453.3334475679162, "Rn/Rc ratio"=26.172570429531696}, {"Rn"=38095.225138873386, "Rc"=1816.3025394885215, "Rn/Rc ratio"=20.97405267604876}, {"Rn"=36531.31136004366, "Rc"=1760.6270814448646, "Rn/Rc ratio"=20.74903410554387}, {"Rn"=36578.86822289468, "Rc"=1701.4405166900585, "Rn/Rc ratio"=21.498764055562948}, {"Rn"=36599.55345425167, "Rc"=1561.5984824041604, "Rn/Rc ratio"=23.437236822812988}, {"Rn"=35081.41992085903, "Rc"=1659.5857768438234, "Rn/Rc ratio"=21.138660267127847}, {"Rn"=34951.13934360826, "Rc"=1838.292643232205, "Rn/Rc ratio"=19.012826642310284}, {"Rn"=35064.70338992991, "Rc"=1726.0321709698853, "Rn/Rc ratio"=20.315208476228165}, {"Rn"=33575.59204648786, "Rc"=1664.5117798461024, "Rn/Rc ratio"=20.17143552423053}, {"Rn"=33563.37385832738, "Rc"=1721.1265727861423, "Rn/Rc ratio"=19.500816726102446}, {"Rn"=33595.894757014525, "Rc"=1931.9089678605308, "Rn/Rc ratio"=17.38999886429426}, {"Rn"=32009.089531727954, "Rc"=1723.8964993278653, "Rn/Rc ratio"=18.567871994756104}, {"Rn"=31838.403083063444, "Rc"=1860.9728516422624, "Rn/Rc ratio"=17.10847262224532}, {"Rn"=32054.10631879645, "Rc"=1478.9784687668719, "Rn/Rc ratio"=21.673139261805623}, {"Rn"=30568.45862557758, "Rc"=1711.399746098411, "Rn/Rc ratio"=17.861670656003355}, {"Rn"=30363.796921054032, "Rc"=1697.1705246998808, "Rn/Rc ratio"=17.89083446781131}, {"Rn"=30432.887272503547, "Rc"=1714.5360796990155, "Rn/Rc ratio"=17.7499252613255}, {"Rn"=29045.329515507692, "Rc"=1922.8475105661091, "Rn/Rc ratio"=15.105373336108386}, {"Rn"=28918.162145937058, "Rc"=1548.5943407250452, "Rn/Rc ratio"=18.67381365503228}, {"Rn"=29043.87394065466, "Rc"=1624.9442562137217, "Rn/Rc ratio"=17.87376633357855}, {"Rn"=27599.286973614016, "Rc"=1872.6491582513668, "Rn/Rc ratio"=14.738098085273776}, {"Rn"=27382.606575130092, "Rc"=1955.3891755298591, "Rn/Rc ratio"=14.003660712558728}, {"Rn"=27518.452745745675, "Rc"=1765.8596240559066, "Rn/Rc ratio"=15.583601533705178}, {"Rn"=26199.53503373307, "Rc"=2074.599477602554, "Rn/Rc ratio"=12.628719575312793}, {"Rn"=26223.058762983255, "Rc"=2044.0740651952274, "Rn/Rc ratio"=12.828820251422112}, {"Rn"=26060.366977863792, "Rc"=1934.1118442410536, "Rn/Rc ratio"=13.474074446863176}, {"Rn"=25297.028178890243, "Rc"=2334.1060871805157, "Rn/Rc ratio"=10.837994175940734}, {"Rn"=25238.67572934048, "Rc"=2437.37519403388, "Rn/Rc ratio"=10.35485869845513}, {"Rn"=25118.026603355065, "Rc"=2247.7535339454234, "Rn/Rc ratio"=11.174724552324935}, {"Rn"=24235.609572772588, "Rc"=2239.4401269538853, "Rn/Rc ratio"=10.822173489290009}, {"Rn"=24157.612662080322, "Rc"=2710.5407785514694, "Rn/Rc ratio"=8.912469737861796}, {"Rn"=24116.44785292884, "Rc"=2315.376353078354, "Rn/Rc ratio"=10.415778765670378}, {"Rn"=23586.060713612686, "Rc"=2305.2128322639132, "Rn/Rc ratio"=10.231619563929456}, {"Rn"=23488.424859310595, "Rc"=2322.9926488914643, "Rn/Rc ratio"=10.11127816978642}, {"Rn"=23574.340363193343, "Rc"=2329.8952487412785, "Rn/Rc ratio"=10.11819753524513}]
  out "dV-dI and Ic Clusters":T1(array[cluster])=[{"Ic (+) (A)"=4.6400000000000005e-09, "Ic (-) (A)"=-4.853333333333333e-09, "Ic (average) (A)"=4.746666666666667e-09}, {"Ic (+) (A)"=4.613333333333334e-09, "Ic (-) (A)"=-4.853333333333333e-09, "Ic (average) (A)"=4.7333333333333335e-09}, {"Ic (+) (A)"=4.506666666666668e-09, "Ic (-) (A)"=-4.906666666666667e-09, "Ic (average) (A)"=4.706666666666668e-09}, {"Ic (+) (A)"=4.693333333333334e-09, "Ic (-) (A)"=-4.906666666666667e-09, "Ic (average) (A)"=4.8e-09}, {"Ic (+) (A)"=4.6400000000000005e-09, "Ic (-) (A)"=-4.906666666666667e-09, "Ic (average) (A)"=4.773333333333333e-09}, {"Ic (+) (A)"=4.72e-09, "Ic (-) (A)"=-4.933333333333334e-09, "Ic (average) (A)"=4.8266666666666665e-09}, {"Ic (+) (A)"=4.746666666666667e-09, "Ic (-) (A)"=-4.88e-09, "Ic (average) (A)"=4.813333333333333e-09}, {"Ic (+) (A)"=4.746666666666667e-09, "Ic (-) (A)"=-4.986666666666667e-09, "Ic (average) (A)"=4.866666666666667e-09}, {"Ic (+) (A)"=4.8e-09, "Ic (-) (A)"=-5.013333333333334e-09, "Ic (average) (A)"=4.906666666666667e-09}, {"Ic (+) (A)"=4.773333333333333e-09, "Ic (-) (A)"=-5.093333333333334e-09, "Ic (average) (A)"=4.933333333333334e-09}, {"Ic (+) (A)"=4.773333333333333e-09, "Ic (-) (A)"=-5.066666666666667e-09, "Ic (average) (A)"=4.92e-09}, {"Ic (+) (A)"=4.8266666666666665e-09, "Ic (-) (A)"=-5.040000000000001e-09, "Ic (average) (A)"=4.933333333333334e-09}, {"Ic (+) (A)"=4.853333333333333e-09, "Ic (-) (A)"=-5.040000000000001e-09, "Ic (average) (A)"=4.946666666666667e-09}, {"Ic (+) (A)"=4.88e-09, "Ic (-) (A)"=-5.040000000000001e-09, "Ic (average) (A)"=4.96e-09}, {"Ic (+) (A)"=4.88e-09, "Ic (-) (A)"=-5.1200000000000005e-09, "Ic (average) (A)"=5e-09}, {"Ic (+) (A)"=5.813333333333333e-09, "Ic (-) (A)"=-5.093333333333334e-09, "Ic (average) (A)"=5.4533333333333335e-09}, {"Ic (+) (A)"=4.88e-09, "Ic (-) (A)"=-5.2e-09, "Ic (average) (A)"=5.04e-09}, {"Ic (+) (A)"=4.960000000000001e-09, "Ic (-) (A)"=-5.2e-09, "Ic (average) (A)"=5.080000000000001e-09}, {"Ic (+) (A)"=4.906666666666666e-09, "Ic (-) (A)"=-5.253333333333333e-09, "Ic (average) (A)"=5.08e-09}, {"Ic (+) (A)"=5.040000000000001e-09, "Ic (-) (A)"=-5.226666666666667e-09, "Ic (average) (A)"=5.133333333333334e-09}, {"Ic (+) (A)"=5.066666666666667e-09, "Ic (-) (A)"=-5.2e-09, "Ic (average) (A)"=5.133333333333334e-09}, {"Ic (+) (A)"=5.1200000000000005e-09, "Ic (-) (A)"=-5.253333333333333e-09, "Ic (average) (A)"=5.186666666666667e-09}, {"Ic (+) (A)"=5.093333333333334e-09, "Ic (-) (A)"=-5.3066666666666665e-09, "Ic (average) (A)"=5.2e-09}, {"Ic (+) (A)"=5.1200000000000005e-09, "Ic (-) (A)"=-5.3066666666666665e-09, "Ic (average) (A)"=5.2133333333333335e-09}, {"Ic (+) (A)"=5.066666666666667e-09, "Ic (-) (A)"=-5.386666666666667e-09, "Ic (average) (A)"=5.226666666666667e-09}, {"Ic (+) (A)"=5.173333333333334e-09, "Ic (-) (A)"=-5.333333333333333e-09, "Ic (average) (A)"=5.253333333333333e-09}, {"Ic (+) (A)"=5.173333333333334e-09, "Ic (-) (A)"=-5.3600000000000005e-09, "Ic (average) (A)"=5.2666666666666675e-09}, {"Ic (+) (A)"=5.253333333333333e-09, "Ic (-) (A)"=-5.413333333333334e-09, "Ic (average) (A)"=5.333333333333333e-09}, {"Ic (+) (A)"=5.2e-09, "Ic (-) (A)"=-5.520000000000001e-09, "Ic (average) (A)"=5.3600000000000005e-09}, {"Ic (+) (A)"=5.28e-09, "Ic (-) (A)"=-5.413333333333334e-09, "Ic (average) (A)"=5.346666666666667e-09}, {"Ic (+) (A)"=5.28e-09, "Ic (-) (A)"=-5.44e-09, "Ic (average) (A)"=5.36e-09}, {"Ic (+) (A)"=5.36e-09, "Ic (-) (A)"=-5.493333333333334e-09, "Ic (average) (A)"=5.426666666666667e-09}, {"Ic (+) (A)"=5.440000000000001e-09, "Ic (-) (A)"=-5.546666666666667e-09, "Ic (average) (A)"=5.493333333333334e-09}, {"Ic (+) (A)"=5.440000000000001e-09, "Ic (-) (A)"=-5.573333333333334e-09, "Ic (average) (A)"=5.5066666666666675e-09}, {"Ic (+) (A)"=5.440000000000001e-09, "Ic (-) (A)"=-5.6000000000000005e-09, "Ic (average) (A)"=5.520000000000001e-09}, {"Ic (+) (A)"=5.440000000000001e-09, "Ic (-) (A)"=-5.706666666666667e-09, "Ic (average) (A)"=5.573333333333334e-09}, {"Ic (+) (A)"=5.466666666666668e-09, "Ic (-) (A)"=-5.733333333333333e-09, "Ic (average) (A)"=5.6000000000000005e-09}, {"Ic (+) (A)"=5.6000000000000005e-09, "Ic (-) (A)"=-5.8400000000000005e-09, "Ic (average) (A)"=5.720000000000001e-09}, {"Ic (+) (A)"=5.520000000000001e-09, "Ic (-) (A)"=-5.7866666666666665e-09, "Ic (average) (A)"=5.653333333333334e-09}, {"Ic (+) (A)"=5.573333333333334e-09, "Ic (-) (A)"=-5.8400000000000005e-09, "Ic (average) (A)"=5.706666666666667e-09}, {"Ic (+) (A)"=5.626666666666667e-09, "Ic (-) (A)"=-5.76e-09, "Ic (average) (A)"=5.6933333333333335e-09}, {"Ic (+) (A)"=5.546666666666667e-09, "Ic (-) (A)"=-5.92e-09, "Ic (average) (A)"=5.733333333333333e-09}, {"Ic (+) (A)"=5.6000000000000005e-09, "Ic (-) (A)"=-5.946666666666668e-09, "Ic (average) (A)"=5.773333333333334e-09}, {"Ic (+) (A)"=5.653333333333334e-09, "Ic (-) (A)"=-5.946666666666668e-09, "Ic (average) (A)"=5.800000000000001e-09}, {"Ic (+) (A)"=5.733333333333333e-09, "Ic (-) (A)"=-5.973333333333334e-09, "Ic (average) (A)"=5.853333333333334e-09}, {"Ic (+) (A)"=5.813333333333333e-09, "Ic (-) (A)"=-6.0800000000000005e-09, "Ic (average) (A)"=5.946666666666667e-09}, {"Ic (+) (A)"=5.866666666666666e-09, "Ic (-) (A)"=-5.973333333333334e-09, "Ic (average) (A)"=5.92e-09}, {"Ic (+) (A)"=5.946666666666668e-09, "Ic (-) (A)"=-6.0800000000000005e-09, "Ic (average) (A)"=6.013333333333334e-09}, {"Ic (+) (A)"=5.946666666666668e-09, "Ic (-) (A)"=-6.0800000000000005e-09, "Ic (average) (A)"=6.013333333333334e-09}, {"Ic (+) (A)"=5.973333333333334e-09, "Ic (-) (A)"=-6.0800000000000005e-09, "Ic (average) (A)"=6.026666666666667e-09}, {"Ic (+) (A)"=5.973333333333334e-09, "Ic (-) (A)"=-6.106666666666667e-09, "Ic (average) (A)"=6.040000000000001e-09}, {"Ic (+) (A)"=5.973333333333334e-09, "Ic (-) (A)"=-6.213333333333333e-09, "Ic (average) (A)"=6.093333333333334e-09}, {"Ic (+) (A)"=5.946666666666668e-09, "Ic (-) (A)"=-6.266666666666667e-09, "Ic (average) (A)"=6.106666666666667e-09}, {"Ic (+) (A)"=6.0800000000000005e-09, "Ic (-) (A)"=-6.16e-09, "Ic (average) (A)"=6.12e-09}, {"Ic (+) (A)"=6.0800000000000005e-09, "Ic (-) (A)"=-6.293333333333334e-09, "Ic (average) (A)"=6.186666666666667e-09}, {"Ic (+) (A)"=6.053333333333334e-09, "Ic (-) (A)"=-6.266666666666667e-09, "Ic (average) (A)"=6.16e-09}, {"Ic (+) (A)"=6.106666666666667e-09, "Ic (-) (A)"=-6.24e-09, "Ic (average) (A)"=6.1733333333333335e-09}, {"Ic (+) (A)"=6.0800000000000005e-09, "Ic (-) (A)"=-6.3200000000000005e-09, "Ic (average) (A)"=6.200000000000001e-09}, {"Ic (+) (A)"=6.186666666666667e-09, "Ic (-) (A)"=-6.426666666666667e-09, "Ic (average) (A)"=6.306666666666667e-09}, {"Ic (+) (A)"=6.133333333333334e-09, "Ic (-) (A)"=-6.346666666666667e-09, "Ic (average) (A)"=6.24e-09}, {"Ic (+) (A)"=6.16e-09, "Ic (-) (A)"=-6.506666666666667e-09, "Ic (average) (A)"=6.333333333333334e-09}, {"Ic (+) (A)"=6.213333333333333e-09, "Ic (-) (A)"=-6.506666666666667e-09, "Ic (average) (A)"=6.36e-09}, {"Ic (+) (A)"=6.32e-09, "Ic (-) (A)"=-6.426666666666667e-09, "Ic (average) (A)"=6.373333333333333e-09}, {"Ic (+) (A)"=6.213333333333333e-09, "Ic (-) (A)"=-6.480000000000001e-09, "Ic (average) (A)"=6.346666666666667e-09}, {"Ic (+) (A)"=6.2666666666666665e-09, "Ic (-) (A)"=-6.453333333333334e-09, "Ic (average) (A)"=6.36e-09}, {"Ic (+) (A)"=6.293333333333333e-09, "Ic (-) (A)"=-6.453333333333334e-09, "Ic (average) (A)"=6.373333333333334e-09}, {"Ic (+) (A)"=6.32e-09, "Ic (-) (A)"=-6.480000000000001e-09, "Ic (average) (A)"=6.4e-09}, {"Ic (+) (A)"=6.400000000000001e-09, "Ic (-) (A)"=-6.453333333333334e-09, "Ic (average) (A)"=6.426666666666668e-09}, {"Ic (+) (A)"=6.293333333333333e-09, "Ic (-) (A)"=-6.480000000000001e-09, "Ic (average) (A)"=6.386666666666667e-09}, {"Ic (+) (A)"=6.400000000000001e-09, "Ic (-) (A)"=-6.613333333333334e-09, "Ic (average) (A)"=6.506666666666667e-09}, {"Ic (+) (A)"=6.426666666666668e-09, "Ic (-) (A)"=-6.64e-09, "Ic (average) (A)"=6.533333333333334e-09}, {"Ic (+) (A)"=6.426666666666668e-09, "Ic (-) (A)"=-6.533333333333334e-09, "Ic (average) (A)"=6.480000000000001e-09}, {"Ic (+) (A)"=6.346666666666666e-09, "Ic (-) (A)"=-6.72e-09, "Ic (average) (A)"=6.533333333333333e-09}, {"Ic (+) (A)"=6.453333333333334e-09, "Ic (-) (A)"=-6.666666666666667e-09, "Ic (average) (A)"=6.5600000000000005e-09}, {"Ic (+) (A)"=6.480000000000001e-09, "Ic (-) (A)"=-6.693333333333333e-09, "Ic (average) (A)"=6.586666666666667e-09}, {"Ic (+) (A)"=6.480000000000001e-09, "Ic (-) (A)"=-6.693333333333333e-09, "Ic (average) (A)"=6.586666666666667e-09}, {"Ic (+) (A)"=6.506666666666667e-09, "Ic (-) (A)"=-6.693333333333333e-09, "Ic (average) (A)"=6.6e-09}, {"Ic (+) (A)"=6.5600000000000005e-09, "Ic (-) (A)"=-6.746666666666667e-09, "Ic (average) (A)"=6.653333333333334e-09}, {"Ic (+) (A)"=6.506666666666667e-09, "Ic (-) (A)"=-6.72e-09, "Ic (average) (A)"=6.613333333333334e-09}, {"Ic (+) (A)"=6.533333333333334e-09, "Ic (-) (A)"=-6.773333333333334e-09, "Ic (average) (A)"=6.653333333333334e-09}, {"Ic (+) (A)"=-8e-09, "Ic (-) (A)"=6.933333333333334e-09, "Ic (average) (A)"=7.466666666666667e-09}, {"Ic (+) (A)"=6.533333333333334e-09, "Ic (-) (A)"=-6.933333333333334e-09, "Ic (average) (A)"=6.733333333333334e-09}, {"Ic (+) (A)"=6.826666666666666e-09, "Ic (-) (A)"=-7.093333333333334e-09, "Ic (average) (A)"=6.96e-09}, {"Ic (+) (A)"=6.773333333333333e-09, "Ic (-) (A)"=-7.013333333333334e-09, "Ic (average) (A)"=6.8933333333333335e-09}, {"Ic (+) (A)"=6.693333333333333e-09, "Ic (-) (A)"=-7.013333333333334e-09, "Ic (average) (A)"=6.853333333333334e-09}, {"Ic (+) (A)"=6.773333333333333e-09, "Ic (-) (A)"=-6.986666666666667e-09, "Ic (average) (A)"=6.88e-09}, {"Ic (+) (A)"=6.8e-09, "Ic (-) (A)"=-7.013333333333334e-09, "Ic (average) (A)"=6.906666666666667e-09}, {"Ic (+) (A)"=6.773333333333333e-09, "Ic (-) (A)"=-7.013333333333334e-09, "Ic (average) (A)"=6.8933333333333335e-09}, {"Ic (+) (A)"=6.7466666666666665e-09, "Ic (-) (A)"=-6.986666666666667e-09, "Ic (average) (A)"=6.866666666666667e-09}, {"Ic (+) (A)"=6.773333333333333e-09, "Ic (-) (A)"=-7.013333333333334e-09, "Ic (average) (A)"=6.8933333333333335e-09}, {"Ic (+) (A)"=6.8e-09, "Ic (-) (A)"=-6.986666666666667e-09, "Ic (average) (A)"=6.8933333333333335e-09}, {"Ic (+) (A)"=6.773333333333333e-09, "Ic (-) (A)"=-6.960000000000001e-09, "Ic (average) (A)"=6.866666666666667e-09}, {"Ic (+) (A)"=6.773333333333333e-09, "Ic (-) (A)"=-6.960000000000001e-09, "Ic (average) (A)"=6.866666666666667e-09}, {"Ic (+) (A)"=6.773333333333333e-09, "Ic (-) (A)"=-6.906666666666667e-09, "Ic (average) (A)"=6.84e-09}, {"Ic (+) (A)"=6.8e-09, "Ic (-) (A)"=-6.933333333333334e-09, "Ic (average) (A)"=6.866666666666667e-09}, {"Ic (+) (A)"=6.8e-09, "Ic (-) (A)"=-6.933333333333334e-09, "Ic (average) (A)"=6.866666666666667e-09}, {"Ic (+) (A)"=6.7466666666666665e-09, "Ic (-) (A)"=-6.960000000000001e-09, "Ic (average) (A)"=6.853333333333334e-09}, {"Ic (+) (A)"=6.773333333333333e-09, "Ic (-) (A)"=-6.986666666666667e-09, "Ic (average) (A)"=6.88e-09}, {"Ic (+) (A)"=6.7466666666666665e-09, "Ic (-) (A)"=-6.960000000000001e-09, "Ic (average) (A)"=6.853333333333334e-09}, {"Ic (+) (A)"=6.826666666666666e-09, "Ic (-) (A)"=-6.933333333333334e-09, "Ic (average) (A)"=6.88e-09}, {"Ic (+) (A)"=6.8e-09, "Ic (-) (A)"=-7.013333333333334e-09, "Ic (average) (A)"=6.906666666666667e-09}, {"Ic (+) (A)"=6.8e-09, "Ic (-) (A)"=-7.0400000000000005e-09, "Ic (average) (A)"=6.92e-09}, {"Ic (+) (A)"=-8e-09, "Ic (-) (A)"=6.773333333333333e-09, "Ic (average) (A)"=7.386666666666667e-09}, {"Ic (+) (A)"=-8e-09, "Ic (-) (A)"=6.8533333333333345e-09, "Ic (average) (A)"=7.4266666666666675e-09}, {"Ic (+) (A)"=0.0, "Ic (-) (A)"=0.0, "Ic (average) (A)"=0.0}, {"Ic (+) (A)"=0.0, "Ic (-) (A)"=0.0, "Ic (average) (A)"=0.0}, {"Ic (+) (A)"=0.0, "Ic (-) (A)"=0.0, "Ic (average) (A)"=0.0}, {"Ic (+) (A)"=0.0, "Ic (-) (A)"=0.0, "Ic (average) (A)"=0.0}, {"Ic (+) (A)"=0.0, "Ic (-) (A)"=0.0, "Ic (average) (A)"=0.0}, {"Ic (+) (A)"=0.0, "Ic (-) (A)"=0.0, "Ic (average) (A)"=0.0}, {"Ic (+) (A)"=0.0, "Ic (-) (A)"=0.0, "Ic (average) (A)"=0.0}, {"Ic (+) (A)"=0.0, "Ic (-) (A)"=0.0, "Ic (average) (A)"=0.0}, {"Ic (+) (A)"=0.0, "Ic (-) (A)"=0.0, "Ic (average) (A)"=0.0}, {"Ic (+) (A)"=0.0, "Ic (-) (A)"=0.0, "Ic (average) (A)"=0.0}, {"Ic (+) (A)"=0.0, "Ic (-) (A)"=0.0, "Ic (average) (A)"=0.0}, {"Ic (+) (A)"=0.0, "Ic (-) (A)"=0.0, "Ic (average) (A)"=0.0}, {"Ic (+) (A)"=0.0, "Ic (-) (A)"=0.0, "Ic (average) (A)"=0.0}, {"Ic (+) (A)"=0.0, "Ic (-) (A)"=0.0, "Ic (average) (A)"=0.0}, {"Ic (+) (A)"=0.0, "Ic (-) (A)"=0.0, "Ic (average) (A)"=0.0}, {"Ic (+) (A)"=0.0, "Ic (-) (A)"=0.0, "Ic (average) (A)"=0.0}, {"Ic (+) (A)"=0.0, "Ic (-) (A)"=0.0, "Ic (average) (A)"=0.0}, {"Ic (+) (A)"=0.0, "Ic (-) (A)"=0.0, "Ic (average) (A)"=0.0}, {"Ic (+) (A)"=0.0, "Ic (-) (A)"=0.0, "Ic (average) (A)"=0.0}, {"Ic (+) (A)"=0.0, "Ic (-) (A)"=0.0, "Ic (average) (A)"=0.0}, {"Ic (+) (A)"=0.0, "Ic (-) (A)"=0.0, "Ic (average) (A)"=0.0}, {"Ic (+) (A)"=0.0, "Ic (-) (A)"=0.0, "Ic (average) (A)"=0.0}, {"Ic (+) (A)"=0.0, "Ic (-) (A)"=0.0, "Ic (average) (A)"=0.0}, {"Ic (+) (A)"=0.0, "Ic (-) (A)"=0.0, "Ic (average) (A)"=0.0}, {"Ic (+) (A)"=0.0, "Ic (-) (A)"=0.0, "Ic (average) (A)"=0.0}, {"Ic (+) (A)"=0.0, "Ic (-) (A)"=0.0, "Ic (average) (A)"=0.0}, {"Ic (+) (A)"=0.0, "Ic (-) (A)"=0.0, "Ic (average) (A)"=0.0}, {"Ic (+) (A)"=0.0, "Ic (-) (A)"=0.0, "Ic (average) (A)"=0.0}, {"Ic (+) (A)"=0.0, "Ic (-) (A)"=0.0, "Ic (average) (A)"=0.0}, {"Ic (+) (A)"=0.0, "Ic (-) (A)"=0.0, "Ic (average) (A)"=0.0}, {"Ic (+) (A)"=0.0, "Ic (-) (A)"=0.0, "Ic (average) (A)"=0.0}, {"Ic (+) (A)"=0.0, "Ic (-) (A)"=0.0, "Ic (average) (A)"=0.0}, {"Ic (+) (A)"=0.0, "Ic (-) (A)"=0.0, "Ic (average) (A)"=0.0}, {"Ic (+) (A)"=0.0, "Ic (-) (A)"=0.0, "Ic (average) (A)"=0.0}, {"Ic (+) (A)"=0.0, "Ic (-) (A)"=0.0, "Ic (average) (A)"=0.0}, {"Ic (+) (A)"=0.0, "Ic (-) (A)"=0.0, "Ic (average) (A)"=0.0}, {"Ic (+) (A)"=0.0, "Ic (-) (A)"=0.0, "Ic (average) (A)"=0.0}, {"Ic (+) (A)"=0.0, "Ic (-) (A)"=0.0, "Ic (average) (A)"=0.0}, {"Ic (+) (A)"=0.0, "Ic (-) (A)"=0.0, "Ic (average) (A)"=0.0}, {"Ic (+) (A)"=0.0, "Ic (-) (A)"=0.0, "Ic (average) (A)"=0.0}, {"Ic (+) (A)"=0.0, "Ic (-) (A)"=0.0, "Ic (average) (A)"=0.0}, {"Ic (+) (A)"=0.0, "Ic (-) (A)"=0.0, "Ic (average) (A)"=0.0}, {"Ic (+) (A)"=0.0, "Ic (-) (A)"=0.0, "Ic (average) (A)"=0.0}, {"Ic (+) (A)"=0.0, "Ic (-) (A)"=0.0, "Ic (average) (A)"=0.0}, {"Ic (+) (A)"=0.0, "Ic (-) (A)"=0.0, "Ic (average) (A)"=0.0}, {"Ic (+) (A)"=0.0, "Ic (-) (A)"=0.0, "Ic (average) (A)"=0.0}, {"Ic (+) (A)"=0.0, "Ic (-) (A)"=0.0, "Ic (average) (A)"=0.0}, {"Ic (+) (A)"=0.0, "Ic (-) (A)"=0.0, "Ic (average) (A)"=0.0}, {"Ic (+) (A)"=0.0, "Ic (-) (A)"=0.0, "Ic (average) (A)"=0.0}, {"Ic (+) (A)"=0.0, "Ic (-) (A)"=0.0, "Ic (average) (A)"=0.0}, {"Ic (+) (A)"=0.0, "Ic (-) (A)"=0.0, "Ic (average) (A)"=0.0}, {"Ic (+) (A)"=0.0, "Ic (-) (A)"=0.0, "Ic (average) (A)"=0.0}, {"Ic (+) (A)"=0.0, "Ic (-) (A)"=0.0, "Ic (average) (A)"=0.0}, {"Ic (+) (A)"=0.0, "Ic (-) (A)"=0.0, "Ic (average) (A)"=0.0}, {"Ic (+) (A)"=0.0, "Ic (-) (A)"=0.0, "Ic (average) (A)"=0.0}, {"Ic (+) (A)"=0.0, "Ic (-) (A)"=0.0, "Ic (average) (A)"=0.0}, {"Ic (+) (A)"=0.0, "Ic (-) (A)"=0.0, "Ic (average) (A)"=0.0}, {"Ic (+) (A)"=0.0, "Ic (-) (A)"=0.0, "Ic (average) (A)"=0.0}, {"Ic (+) (A)"=6.8533333333333345e-09, "Ic (-) (A)"=-7.013333333333334e-09, "Ic (average) (A)"=6.933333333333334e-09}, {"Ic (+) (A)"=6.826666666666666e-09, "Ic (-) (A)"=-7.013333333333334e-09, "Ic (average) (A)"=6.92e-09}, {"Ic (+) (A)"=6.8e-09, "Ic (-) (A)"=-6.986666666666667e-09, "Ic (average) (A)"=6.8933333333333335e-09}, {"Ic (+) (A)"=6.826666666666666e-09, "Ic (-) (A)"=-6.960000000000001e-09, "Ic (average) (A)"=6.8933333333333335e-09}, {"Ic (+) (A)"=6.773333333333333e-09, "Ic (-) (A)"=-6.960000000000001e-09, "Ic (average) (A)"=6.866666666666667e-09}, {"Ic (+) (A)"=6.7466666666666665e-09, "Ic (-) (A)"=-6.960000000000001e-09, "Ic (average) (A)"=6.853333333333334e-09}, {"Ic (+) (A)"=6.5600000000000005e-09, "Ic (-) (A)"=-7.0400000000000005e-09, "Ic (average) (A)"=6.8000000000000005e-09}, {"Ic (+) (A)"=6.586666666666667e-09, "Ic (-) (A)"=-6.960000000000001e-09, "Ic (average) (A)"=6.773333333333334e-09}, {"Ic (+) (A)"=6.613333333333334e-09, "Ic (-) (A)"=-6.773333333333334e-09, "Ic (average) (A)"=6.693333333333333e-09}, {"Ic (+) (A)"=6.480000000000001e-09, "Ic (-) (A)"=-6.666666666666667e-09, "Ic (average) (A)"=6.573333333333334e-09}, {"Ic (+) (A)"=6.426666666666668e-09, "Ic (-) (A)"=-6.666666666666667e-09, "Ic (average) (A)"=6.546666666666667e-09}, {"Ic (+) (A)"=6.453333333333334e-09, "Ic (-) (A)"=-6.666666666666667e-09, "Ic (average) (A)"=6.5600000000000005e-09}, {"Ic (+) (A)"=6.213333333333333e-09, "Ic (-) (A)"=-6.426666666666667e-09, "Ic (average) (A)"=6.32e-09}, {"Ic (+) (A)"=6.213333333333333e-09, "Ic (-) (A)"=-6.533333333333334e-09, "Ic (average) (A)"=6.373333333333334e-09}, {"Ic (+) (A)"=6.293333333333333e-09, "Ic (-) (A)"=-6.426666666666667e-09, "Ic (average) (A)"=6.36e-09}, {"Ic (+) (A)"=6.133333333333334e-09, "Ic (-) (A)"=-6.186666666666667e-09, "Ic (average) (A)"=6.16e-09}, {"Ic (+) (A)"=6.0800000000000005e-09, "Ic (-) (A)"=-6.24e-09, "Ic (average) (A)"=6.16e-09}, {"Ic (+) (A)"=6.0800000000000005e-09, "Ic (-) (A)"=-6.24e-09, "Ic (average) (A)"=6.16e-09}, {"Ic (+) (A)"=6.000000000000001e-09, "Ic (-) (A)"=-6.106666666666667e-09, "Ic (average) (A)"=6.053333333333334e-09}, {"Ic (+) (A)"=5.973333333333334e-09, "Ic (-) (A)"=-6.106666666666667e-09, "Ic (average) (A)"=6.040000000000001e-09}, {"Ic (+) (A)"=5.8933333333333345e-09, "Ic (-) (A)"=-6.106666666666667e-09, "Ic (average) (A)"=6.000000000000001e-09}, {"Ic (+) (A)"=5.706666666666667e-09, "Ic (-) (A)"=-5.893333333333334e-09, "Ic (average) (A)"=5.800000000000001e-09}, {"Ic (+) (A)"=5.76e-09, "Ic (-) (A)"=-5.8400000000000005e-09, "Ic (average) (A)"=5.800000000000001e-09}, {"Ic (+) (A)"=5.68e-09, "Ic (-) (A)"=-5.7866666666666665e-09, "Ic (average) (A)"=5.733333333333333e-09}, {"Ic (+) (A)"=5.493333333333334e-09, "Ic (-) (A)"=-5.626666666666667e-09, "Ic (average) (A)"=5.560000000000001e-09}, {"Ic (+) (A)"=5.520000000000001e-09, "Ic (-) (A)"=-5.653333333333334e-09, "Ic (average) (A)"=5.586666666666667e-09}, {"Ic (+) (A)"=5.546666666666667e-09, "Ic (-) (A)"=-5.733333333333333e-09, "Ic (average) (A)"=5.64e-09}, {"Ic (+) (A)"=5.3066666666666665e-09, "Ic (-) (A)"=-5.44e-09, "Ic (average) (A)"=5.373333333333334e-09}, {"Ic (+) (A)"=5.333333333333333e-09, "Ic (-) (A)"=-5.44e-09, "Ic (average) (A)"=5.386666666666666e-09}, {"Ic (+) (A)"=5.28e-09, "Ic (-) (A)"=-5.466666666666667e-09, "Ic (average) (A)"=5.373333333333334e-09}, {"Ic (+) (A)"=5.2e-09, "Ic (-) (A)"=-5.3066666666666665e-09, "Ic (average) (A)"=5.253333333333333e-09}, {"Ic (+) (A)"=5.253333333333333e-09, "Ic (-) (A)"=-5.3600000000000005e-09, "Ic (average) (A)"=5.3066666666666665e-09}, {"Ic (+) (A)"=5.2e-09, "Ic (-) (A)"=-5.386666666666667e-09, "Ic (average) (A)"=5.293333333333334e-09}, {"Ic (+) (A)"=5.1200000000000005e-09, "Ic (-) (A)"=-5.3066666666666665e-09, "Ic (average) (A)"=5.2133333333333335e-09}, {"Ic (+) (A)"=5.093333333333334e-09, "Ic (-) (A)"=-5.253333333333333e-09, "Ic (average) (A)"=5.173333333333334e-09}, {"Ic (+) (A)"=5.040000000000001e-09, "Ic (-) (A)"=-5.3066666666666665e-09, "Ic (average) (A)"=5.173333333333334e-09}, {"Ic (+) (A)"=4.88e-09, "Ic (-) (A)"=-5.146666666666667e-09, "Ic (average) (A)"=5.013333333333333e-09}, {"Ic (+) (A)"=4.906666666666666e-09, "Ic (-) (A)"=-5.146666666666667e-09, "Ic (average) (A)"=5.026666666666667e-09}, {"Ic (+) (A)"=5.013333333333334e-09, "Ic (-) (A)"=-5.173333333333334e-09, "Ic (average) (A)"=5.093333333333334e-09}, {"Ic (+) (A)"=4.8e-09, "Ic (-) (A)"=-5.013333333333334e-09, "Ic (average) (A)"=4.906666666666667e-09}, {"Ic (+) (A)"=4.8e-09, "Ic (-) (A)"=-5.040000000000001e-09, "Ic (average) (A)"=4.92e-09}, {"Ic (+) (A)"=4.853333333333333e-09, "Ic (-) (A)"=-5.066666666666667e-09, "Ic (average) (A)"=4.96e-09}, {"Ic (+) (A)"=4.746666666666667e-09, "Ic (-) (A)"=-4.933333333333334e-09, "Ic (average) (A)"=4.840000000000001e-09}, {"Ic (+) (A)"=4.773333333333333e-09, "Ic (-) (A)"=-4.933333333333334e-09, "Ic (average) (A)"=4.853333333333333e-09}, {"Ic (+) (A)"=4.773333333333333e-09, "Ic (-) (A)"=-4.933333333333334e-09, "Ic (average) (A)"=4.853333333333333e-09}, {"Ic (+) (A)"=4.693333333333334e-09, "Ic (-) (A)"=-4.853333333333333e-09, "Ic (average) (A)"=4.773333333333333e-09}, {"Ic (+) (A)"=4.613333333333334e-09, "Ic (-) (A)"=-4.906666666666667e-09, "Ic (average) (A)"=4.760000000000001e-09}, {"Ic (+) (A)"=4.666666666666667e-09, "Ic (-) (A)"=-4.853333333333333e-09, "Ic (average) (A)"=4.76e-09}, {"Ic (+) (A)"=4.613333333333334e-09, "Ic (-) (A)"=-4.72e-09, "Ic (average) (A)"=4.666666666666667e-09}, {"Ic (+) (A)"=4.560000000000001e-09, "Ic (-) (A)"=-4.773333333333333e-09, "Ic (average) (A)"=4.666666666666667e-09}, {"Ic (+) (A)"=4.613333333333334e-09, "Ic (-) (A)"=-4.8266666666666665e-09, "Ic (average) (A)"=4.72e-09}, {"Ic (+) (A)"=4.480000000000001e-09, "Ic (-) (A)"=-4.72e-09, "Ic (average) (A)"=4.600000000000001e-09}, {"Ic (+) (A)"=4.4e-09, "Ic (-) (A)"=-4.6400000000000005e-09, "Ic (average) (A)"=4.52e-09}, {"Ic (+) (A)"=4.4e-09, "Ic (-) (A)"=-4.72e-09, "Ic (average) (A)"=4.56e-09}, {"Ic (+) (A)"=4.426666666666666e-09, "Ic (-) (A)"=-4.533333333333334e-09, "Ic (average) (A)"=4.48e-09}, {"Ic (+) (A)"=4.3466666666666665e-09, "Ic (-) (A)"=-4.506666666666667e-09, "Ic (average) (A)"=4.426666666666666e-09}, {"Ic (+) (A)"=4.373333333333333e-09, "Ic (-) (A)"=-4.586666666666667e-09, "Ic (average) (A)"=4.48e-09}, {"Ic (+) (A)"=4.266666666666667e-09, "Ic (-) (A)"=-4.48e-09, "Ic (average) (A)"=4.373333333333333e-09}, {"Ic (+) (A)"=4.266666666666667e-09, "Ic (-) (A)"=-4.426666666666667e-09, "Ic (average) (A)"=4.3466666666666665e-09}, {"Ic (+) (A)"=4.1600000000000005e-09, "Ic (-) (A)"=-4.453333333333334e-09, "Ic (average) (A)"=4.3066666666666675e-09}, {"Ic (+) (A)"=4.1600000000000005e-09, "Ic (-) (A)"=-4.293333333333333e-09, "Ic (average) (A)"=4.226666666666667e-09}, {"Ic (+) (A)"=4.1600000000000005e-09, "Ic (-) (A)"=-4.3466666666666665e-09, "Ic (average) (A)"=4.2533333333333335e-09}, {"Ic (+) (A)"=4.1600000000000005e-09, "Ic (-) (A)"=-4.32e-09, "Ic (average) (A)"=4.24e-09}, {"Ic (+) (A)"=4.133333333333334e-09, "Ic (-) (A)"=-4.32e-09, "Ic (average) (A)"=4.226666666666667e-09}, {"Ic (+) (A)"=4.080000000000001e-09, "Ic (-) (A)"=-4.3466666666666665e-09, "Ic (average) (A)"=4.213333333333334e-09}, {"Ic (+) (A)"=4.106666666666667e-09, "Ic (-) (A)"=-4.293333333333333e-09, "Ic (average) (A)"=4.2e-09}, {"Ic (+) (A)"=4.053333333333334e-09, "Ic (-) (A)"=-4.24e-09, "Ic (average) (A)"=4.146666666666667e-09}, {"Ic (+) (A)"=4.106666666666667e-09, "Ic (-) (A)"=-4.24e-09, "Ic (average) (A)"=4.173333333333334e-09}, {"Ic (+) (A)"=4.026666666666668e-09, "Ic (-) (A)"=-4.186666666666667e-09, "Ic (average) (A)"=4.106666666666667e-09}, {"Ic (+) (A)"=3.893333333333333e-09, "Ic (-) (A)"=-4.186666666666667e-09, "Ic (average) (A)"=4.04e-09}, {"Ic (+) (A)"=3.893333333333333e-09, "Ic (-) (A)"=-4.053333333333333e-09, "Ic (average) (A)"=3.973333333333333e-09}, {"Ic (+) (A)"=3.893333333333333e-09, "Ic (-) (A)"=-4.986666666666667e-09, "Ic (average) (A)"=4.44e-09}, {"Ic (+) (A)"=3.893333333333333e-09, "Ic (-) (A)"=-4.026666666666667e-09, "Ic (average) (A)"=3.96e-09}, {"Ic (+) (A)"=3.8666666666666665e-09, "Ic (-) (A)"=-4.08e-09, "Ic (average) (A)"=3.973333333333333e-09}, {"Ic (+) (A)"=3.8666666666666665e-09, "Ic (-) (A)"=-4.053333333333333e-09, "Ic (average) (A)"=3.96e-09}, {"Ic (+) (A)"=3.706666666666667e-09, "Ic (-) (A)"=-3.946666666666667e-09, "Ic (average) (A)"=3.8266666666666675e-09}, {"Ic (+) (A)"=3.733333333333334e-09, "Ic (-) (A)"=-3.973333333333334e-09, "Ic (average) (A)"=3.853333333333334e-09}, {"Ic (+) (A)"=3.786666666666667e-09, "Ic (-) (A)"=-4.666666666666667e-09, "Ic (average) (A)"=4.226666666666667e-09}, {"Ic (+) (A)"=3.706666666666667e-09, "Ic (-) (A)"=-3.973333333333334e-09, "Ic (average) (A)"=3.84e-09}, {"Ic (+) (A)"=3.6800000000000005e-09, "Ic (-) (A)"=-3.946666666666667e-09, "Ic (average) (A)"=3.813333333333333e-09}, {"Ic (+) (A)"=3.786666666666667e-09, "Ic (-) (A)"=-3.946666666666667e-09, "Ic (average) (A)"=3.8666666666666665e-09}, {"Ic (+) (A)"=3.6266666666666674e-09, "Ic (-) (A)"=-3.9200000000000005e-09, "Ic (average) (A)"=3.773333333333334e-09}, {"Ic (+) (A)"=3.706666666666667e-09, "Ic (-) (A)"=-3.84e-09, "Ic (average) (A)"=3.7733333333333335e-09}, {"Ic (+) (A)"=3.653333333333334e-09, "Ic (-) (A)"=-3.893333333333334e-09, "Ic (average) (A)"=3.773333333333334e-09}, {"Ic (+) (A)"=3.6266666666666674e-09, "Ic (-) (A)"=-3.893333333333334e-09, "Ic (average) (A)"=3.76e-09}, {"Ic (+) (A)"=3.600000000000001e-09, "Ic (-) (A)"=-3.84e-09, "Ic (average) (A)"=3.7200000000000004e-09}, {"Ic (+) (A)"=3.653333333333334e-09, "Ic (-) (A)"=-3.893333333333334e-09, "Ic (average) (A)"=3.773333333333334e-09}, {"Ic (+) (A)"=3.600000000000001e-09, "Ic (-) (A)"=-3.84e-09, "Ic (average) (A)"=3.7200000000000004e-09}, {"Ic (+) (A)"=3.600000000000001e-09, "Ic (-) (A)"=-3.893333333333334e-09, "Ic (average) (A)"=3.746666666666668e-09}, {"Ic (+) (A)"=3.653333333333334e-09, "Ic (-) (A)"=-3.813333333333333e-09, "Ic (average) (A)"=3.733333333333334e-09}, {"Ic (+) (A)"=3.5466666666666677e-09, "Ic (-) (A)"=-3.733333333333334e-09, "Ic (average) (A)"=3.6400000000000007e-09}, {"Ic (+) (A)"=3.600000000000001e-09, "Ic (-) (A)"=-3.706666666666667e-09, "Ic (average) (A)"=3.653333333333334e-09}, {"Ic (+) (A)"=3.5199999999999994e-09, "Ic (-) (A)"=-3.813333333333333e-09, "Ic (average) (A)"=3.6666666666666664e-09}, {"Ic (+) (A)"=3.5199999999999994e-09, "Ic (-) (A)"=-3.76e-09, "Ic (average) (A)"=3.64e-09}, {"Ic (+) (A)"=3.5199999999999994e-09, "Ic (-) (A)"=-3.733333333333334e-09, "Ic (average) (A)"=3.6266666666666666e-09}, {"Ic (+) (A)"=3.5199999999999994e-09, "Ic (-) (A)"=-3.76e-09, "Ic (average) (A)"=3.64e-09}, {"Ic (+) (A)"=3.413333333333333e-09, "Ic (-) (A)"=-3.6266666666666666e-09, "Ic (average) (A)"=3.52e-09}, {"Ic (+) (A)"=3.3866666666666666e-09, "Ic (-) (A)"=-3.5733333333333334e-09, "Ic (average) (A)"=3.48e-09}, {"Ic (+) (A)"=3.413333333333333e-09, "Ic (-) (A)"=-3.653333333333334e-09, "Ic (average) (A)"=3.5333333333333335e-09}, {"Ic (+) (A)"=3.3333333333333334e-09, "Ic (-) (A)"=-3.5733333333333334e-09, "Ic (average) (A)"=3.4533333333333334e-09}, {"Ic (+) (A)"=3.306666666666667e-09, "Ic (-) (A)"=-3.5200000000000003e-09, "Ic (average) (A)"=3.4133333333333335e-09}, {"Ic (+) (A)"=3.306666666666667e-09, "Ic (-) (A)"=-3.5733333333333334e-09, "Ic (average) (A)"=3.44e-09}, {"Ic (+) (A)"=3.226666666666667e-09, "Ic (-) (A)"=-3.466666666666667e-09, "Ic (average) (A)"=3.346666666666667e-09}, {"Ic (+) (A)"=3.226666666666667e-09, "Ic (-) (A)"=-3.413333333333334e-09, "Ic (average) (A)"=3.3200000000000005e-09}, {"Ic (+) (A)"=3.1466666666666674e-09, "Ic (-) (A)"=-3.4400000000000005e-09, "Ic (average) (A)"=3.293333333333334e-09}, {"Ic (+) (A)"=3.1466666666666674e-09, "Ic (-) (A)"=-3.413333333333334e-09, "Ic (average) (A)"=3.2800000000000007e-09}, {"Ic (+) (A)"=3.1466666666666674e-09, "Ic (-) (A)"=-3.413333333333334e-09, "Ic (average) (A)"=3.2800000000000007e-09}, {"Ic (+) (A)"=3.120000000000001e-09, "Ic (-) (A)"=-3.413333333333334e-09, "Ic (average) (A)"=3.2666666666666674e-09}, {"Ic (+) (A)"=3.0933333333333342e-09, "Ic (-) (A)"=-3.36e-09, "Ic (average) (A)"=3.226666666666667e-09}, {"Ic (+) (A)"=3.013333333333333e-09, "Ic (-) (A)"=-3.3333333333333334e-09, "Ic (average) (A)"=3.173333333333333e-09}, {"Ic (+) (A)"=3.013333333333333e-09, "Ic (-) (A)"=-3.2533333333333337e-09, "Ic (average) (A)"=3.1333333333333333e-09}, {"Ic (+) (A)"=3.0399999999999994e-09, "Ic (-) (A)"=-3.226666666666667e-09, "Ic (average) (A)"=3.1333333333333333e-09}, {"Ic (+) (A)"=2.9599999999999997e-09, "Ic (-) (A)"=-3.226666666666667e-09, "Ic (average) (A)"=3.0933333333333334e-09}, {"Ic (+) (A)"=2.9599999999999997e-09, "Ic (-) (A)"=-3.2533333333333337e-09, "Ic (average) (A)"=3.1066666666666667e-09}, {"Ic (+) (A)"=2.826666666666667e-09, "Ic (-) (A)"=-3.12e-09, "Ic (average) (A)"=2.9733333333333334e-09}, {"Ic (+) (A)"=2.826666666666667e-09, "Ic (-) (A)"=-3.173333333333333e-09, "Ic (average) (A)"=3e-09}, {"Ic (+) (A)"=3.2000000000000005e-09, "Ic (-) (A)"=-3.0133333333333337e-09, "Ic (average) (A)"=3.106666666666667e-09}, {"Ic (+) (A)"=3.0399999999999994e-09, "Ic (-) (A)"=-3.1466666666666666e-09, "Ic (average) (A)"=3.093333333333333e-09}, {"Ic (+) (A)"=2.9599999999999997e-09, "Ic (-) (A)"=-3.5733333333333334e-09, "Ic (average) (A)"=3.2666666666666666e-09}, {"Ic (+) (A)"=2.9066666666666666e-09, "Ic (-) (A)"=-3.2533333333333337e-09, "Ic (average) (A)"=3.08e-09}, {"Ic (+) (A)"=2.826666666666667e-09, "Ic (-) (A)"=-3.0933333333333334e-09, "Ic (average) (A)"=2.96e-09}, {"Ic (+) (A)"=2.7733333333333337e-09, "Ic (-) (A)"=-3.0400000000000003e-09, "Ic (average) (A)"=2.906666666666667e-09}, {"Ic (+) (A)"=2.8000000000000003e-09, "Ic (-) (A)"=-2.9600000000000005e-09, "Ic (average) (A)"=2.8800000000000004e-09}, {"Ic (+) (A)"=2.746666666666667e-09, "Ic (-) (A)"=-2.933333333333333e-09, "Ic (average) (A)"=2.84e-09}, {"Ic (+) (A)"=2.693333333333334e-09, "Ic (-) (A)"=-2.9066666666666666e-09, "Ic (average) (A)"=2.8000000000000003e-09}, {"Ic (+) (A)"=2.7200000000000005e-09, "Ic (-) (A)"=-2.9600000000000005e-09, "Ic (average) (A)"=2.8400000000000005e-09}, {"Ic (+) (A)"=2.586666666666666e-09, "Ic (-) (A)"=-2.8000000000000003e-09, "Ic (average) (A)"=2.693333333333333e-09}, {"Ic (+) (A)"=2.586666666666666e-09, "Ic (-) (A)"=-2.826666666666667e-09, "Ic (average) (A)"=2.7066666666666664e-09}, {"Ic (+) (A)"=2.586666666666666e-09, "Ic (-) (A)"=-2.8000000000000003e-09, "Ic (average) (A)"=2.693333333333333e-09}, {"Ic (+) (A)"=2.4799999999999997e-09, "Ic (-) (A)"=-2.693333333333333e-09, "Ic (average) (A)"=2.5866666666666664e-09}, {"Ic (+) (A)"=2.4266666666666666e-09, "Ic (-) (A)"=-2.693333333333333e-09, "Ic (average) (A)"=2.56e-09}, {"Ic (+) (A)"=2.5066666666666663e-09, "Ic (-) (A)"=-2.693333333333333e-09, "Ic (average) (A)"=2.5999999999999997e-09}, {"Ic (+) (A)"=2.4266666666666666e-09, "Ic (-) (A)"=-2.746666666666667e-09, "Ic (average) (A)"=2.586666666666667e-09}, {"Ic (+) (A)"=2.4e-09, "Ic (-) (A)"=-2.64e-09, "Ic (average) (A)"=2.52e-09}, {"Ic (+) (A)"=2.4e-09, "Ic (-) (A)"=-2.6133333333333334e-09, "Ic (average) (A)"=2.5066666666666667e-09}, {"Ic (+) (A)"=2.346666666666667e-09, "Ic (-) (A)"=-2.5333333333333337e-09, "Ic (average) (A)"=2.4400000000000003e-09}, {"Ic (+) (A)"=2.9599999999999997e-09, "Ic (-) (A)"=-2.4800000000000005e-09, "Ic (average) (A)"=2.72e-09}, {"Ic (+) (A)"=2.266666666666667e-09, "Ic (-) (A)"=-2.586666666666667e-09, "Ic (average) (A)"=2.426666666666667e-09}, {"Ic (+) (A)"=2.160000000000001e-09, "Ic (-) (A)"=-2.5600000000000003e-09, "Ic (average) (A)"=2.3600000000000005e-09}, {"Ic (+) (A)"=2.213333333333334e-09, "Ic (-) (A)"=-2.4800000000000005e-09, "Ic (average) (A)"=2.3466666666666672e-09}, {"Ic (+) (A)"=2.346666666666667e-09, "Ic (-) (A)"=-2.453333333333333e-09, "Ic (average) (A)"=2.4e-09}, {"Ic (+) (A)"=2.213333333333334e-09, "Ic (-) (A)"=-2.3733333333333334e-09, "Ic (average) (A)"=2.2933333333333337e-09}, {"Ic (+) (A)"=2.213333333333334e-09, "Ic (-) (A)"=-2.4266666666666666e-09, "Ic (average) (A)"=2.3200000000000003e-09}, {"Ic (+) (A)"=2.1866666666666674e-09, "Ic (-) (A)"=-2.4e-09, "Ic (average) (A)"=2.2933333333333337e-09}, {"Ic (+) (A)"=2.106666666666666e-09, "Ic (-) (A)"=-2.2933333333333337e-09, "Ic (average) (A)"=2.2e-09}, {"Ic (+) (A)"=2.160000000000001e-09, "Ic (-) (A)"=-2.3733333333333334e-09, "Ic (average) (A)"=2.266666666666667e-09}, {"Ic (+) (A)"=2.1333333333333342e-09, "Ic (-) (A)"=-2.3733333333333334e-09, "Ic (average) (A)"=2.253333333333334e-09}, {"Ic (+) (A)"=2.0799999999999994e-09, "Ic (-) (A)"=-2.4266666666666666e-09, "Ic (average) (A)"=2.253333333333333e-09}, {"Ic (+) (A)"=2.0266666666666663e-09, "Ic (-) (A)"=-2.266666666666667e-09, "Ic (average) (A)"=2.1466666666666667e-09}, {"Ic (+) (A)"=2.1333333333333342e-09, "Ic (-) (A)"=-2.266666666666667e-09, "Ic (average) (A)"=2.2000000000000007e-09}, {"Ic (+) (A)"=2.0799999999999994e-09, "Ic (-) (A)"=-2.346666666666667e-09, "Ic (average) (A)"=2.213333333333333e-09}, {"Ic (+) (A)"=2.053333333333333e-09, "Ic (-) (A)"=-2.2933333333333337e-09, "Ic (average) (A)"=2.1733333333333333e-09}, {"Ic (+) (A)"=2.0799999999999994e-09, "Ic (-) (A)"=-2.2933333333333337e-09, "Ic (average) (A)"=2.1866666666666666e-09}, {"Ic (+) (A)"=2.053333333333333e-09, "Ic (-) (A)"=-2.213333333333333e-09, "Ic (average) (A)"=2.133333333333333e-09}, {"Ic (+) (A)"=1.973333333333333e-09, "Ic (-) (A)"=-2.2400000000000005e-09, "Ic (average) (A)"=2.106666666666667e-09}, {"Ic (+) (A)"=2.053333333333333e-09, "Ic (-) (A)"=-2.346666666666667e-09, "Ic (average) (A)"=2.2e-09}, {"Ic (+) (A)"=1.9466666666666666e-09, "Ic (-) (A)"=-2.4e-09, "Ic (average) (A)"=2.1733333333333333e-09}, {"Ic (+) (A)"=1.9999999999999997e-09, "Ic (-) (A)"=-2.16e-09, "Ic (average) (A)"=2.08e-09}, {"Ic (+) (A)"=1.973333333333333e-09, "Ic (-) (A)"=-2.2933333333333337e-09, "Ic (average) (A)"=2.1333333333333334e-09}, {"Ic (+) (A)"=2.0266666666666663e-09, "Ic (-) (A)"=-2.346666666666667e-09, "Ic (average) (A)"=2.1866666666666666e-09}, {"Ic (+) (A)"=1.866666666666667e-09, "Ic (-) (A)"=-2.1866666666666666e-09, "Ic (average) (A)"=2.0266666666666667e-09}, {"Ic (+) (A)"=1.9999999999999997e-09, "Ic (-) (A)"=-2.16e-09, "Ic (average) (A)"=2.08e-09}, {"Ic (+) (A)"=1.9466666666666666e-09, "Ic (-) (A)"=-2.933333333333333e-09, "Ic (average) (A)"=2.44e-09}, {"Ic (+) (A)"=1.8933333333333334e-09, "Ic (-) (A)"=-2.1333333333333334e-09, "Ic (average) (A)"=2.0133333333333334e-09}, {"Ic (+) (A)"=2.0266666666666663e-09, "Ic (-) (A)"=-2.2933333333333337e-09, "Ic (average) (A)"=2.16e-09}, {"Ic (+) (A)"=1.973333333333333e-09, "Ic (-) (A)"=-2.213333333333333e-09, "Ic (average) (A)"=2.093333333333333e-09}, {"Ic (+) (A)"=1.9466666666666666e-09, "Ic (-) (A)"=-2.2933333333333337e-09, "Ic (average) (A)"=2.12e-09}, {"Ic (+) (A)"=1.8400000000000003e-09, "Ic (-) (A)"=-2.16e-09, "Ic (average) (A)"=2e-09}, {"Ic (+) (A)"=1.9999999999999997e-09, "Ic (-) (A)"=-1.8933333333333334e-09, "Ic (average) (A)"=1.9466666666666666e-09}, {"Ic (+) (A)"=1.9466666666666666e-09, "Ic (-) (A)"=-2.0800000000000003e-09, "Ic (average) (A)"=2.0133333333333334e-09}, {"Ic (+) (A)"=1.8133333333333337e-09, "Ic (-) (A)"=-2.1333333333333334e-09, "Ic (average) (A)"=1.9733333333333335e-09}, {"Ic (+) (A)"=1.973333333333333e-09, "Ic (-) (A)"=-1.92e-09, "Ic (average) (A)"=1.9466666666666666e-09}, {"Ic (+) (A)"=1.8400000000000003e-09, "Ic (-) (A)"=-2.0800000000000003e-09, "Ic (average) (A)"=1.9600000000000003e-09}, {"Ic (+) (A)"=1.7066666666666674e-09, "Ic (-) (A)"=-2.0800000000000003e-09, "Ic (average) (A)"=1.893333333333334e-09}, {"Ic (+) (A)"=1.7066666666666674e-09, "Ic (-) (A)"=-1.2799999999999997e-09, "Ic (average) (A)"=1.4933333333333336e-09}, {"Ic (+) (A)"=1.92e-09, "Ic (-) (A)"=-2.64e-09, "Ic (average) (A)"=2.28e-09}, {"Ic (+) (A)"=1.0933333333333329e-09, "Ic (-) (A)"=-2.0533333333333337e-09, "Ic (average) (A)"=1.5733333333333333e-09}, {"Ic (+) (A)"=2.0266666666666663e-09, "Ic (-) (A)"=-2.0800000000000003e-09, "Ic (average) (A)"=2.0533333333333333e-09}, {"Ic (+) (A)"=1.1199999999999994e-09, "Ic (-) (A)"=-2.106666666666667e-09, "Ic (average) (A)"=1.6133333333333331e-09}, {"Ic (+) (A)"=1.7066666666666674e-09, "Ic (-) (A)"=-1.973333333333333e-09, "Ic (average) (A)"=1.8400000000000003e-09}, {"Ic (+) (A)"=1.733333333333334e-09, "Ic (-) (A)"=-1.5199999999999997e-09, "Ic (average) (A)"=1.6266666666666668e-09}, {"Ic (+) (A)"=1.6800000000000008e-09, "Ic (-) (A)"=-1.8400000000000003e-09, "Ic (average) (A)"=1.7600000000000005e-09}, {"Ic (+) (A)"=1.5999999999999994e-09, "Ic (-) (A)"=-1.5199999999999997e-09, "Ic (average) (A)"=1.5599999999999996e-09}, {"Ic (+) (A)"=1.4666666666666666e-09, "Ic (-) (A)"=-1.3066666666666671e-09, "Ic (average) (A)"=1.3866666666666668e-09}, {"Ic (+) (A)"=1.8133333333333337e-09, "Ic (-) (A)"=-1.8400000000000003e-09, "Ic (average) (A)"=1.826666666666667e-09}, {"Ic (+) (A)"=1.7866666666666671e-09, "Ic (-) (A)"=-2.0800000000000003e-09, "Ic (average) (A)"=1.9333333333333337e-09}, {"Ic (+) (A)"=1.5999999999999994e-09, "Ic (-) (A)"=-9.066666666666668e-10, "Ic (average) (A)"=1.2533333333333331e-09}, {"Ic (+) (A)"=1.626666666666666e-09, "Ic (-) (A)"=-1.8133333333333337e-09, "Ic (average) (A)"=1.7199999999999999e-09}, {"Ic (+) (A)"=1.253333333333334e-09, "Ic (-) (A)"=-1.8133333333333337e-09, "Ic (average) (A)"=1.5333333333333338e-09}, {"Ic (+) (A)"=9.066666666666668e-10, "Ic (-) (A)"=-2.0000000000000005e-09, "Ic (average) (A)"=1.4533333333333337e-09}, {"Ic (+) (A)"=2.1333333333333342e-09, "Ic (-) (A)"=-1.7599999999999997e-09, "Ic (average) (A)"=1.946666666666667e-09}, {"Ic (+) (A)"=1.626666666666666e-09, "Ic (-) (A)"=-2.0533333333333337e-09, "Ic (average) (A)"=1.8399999999999998e-09}, {"Ic (+) (A)"=1.3866666666666668e-09, "Ic (-) (A)"=-1.4933333333333331e-09, "Ic (average) (A)"=1.44e-09}, {"Ic (+) (A)"=1.44e-09, "Ic (-) (A)"=-1.6266666666666668e-09, "Ic (average) (A)"=1.5333333333333334e-09}, {"Ic (+) (A)"=7.466666666666674e-10, "Ic (-) (A)"=-1.973333333333333e-09, "Ic (average) (A)"=1.3600000000000003e-09}, {"Ic (+) (A)"=1.44e-09, "Ic (-) (A)"=-1.92e-09, "Ic (average) (A)"=1.68e-09}, {"Ic (+) (A)"=8.000000000000005e-10, "Ic (-) (A)"=-1.68e-09, "Ic (average) (A)"=1.2400000000000003e-09}, {"Ic (+) (A)"=8.000000000000005e-10, "Ic (-) (A)"=-9.6e-10, "Ic (average) (A)"=8.800000000000003e-10}, {"Ic (+) (A)"=1.4666666666666666e-09, "Ic (-) (A)"=-1.7599999999999997e-09, "Ic (average) (A)"=1.6133333333333331e-09}, {"Ic (+) (A)"=1.5199999999999997e-09, "Ic (-) (A)"=-1.5733333333333337e-09, "Ic (average) (A)"=1.5466666666666667e-09}, {"Ic (+) (A)"=9.066666666666668e-10, "Ic (-) (A)"=-1.6266666666666668e-09, "Ic (average) (A)"=1.2666666666666668e-09}, {"Ic (+) (A)"=1.3866666666666668e-09, "Ic (-) (A)"=-1.7599999999999997e-09, "Ic (average) (A)"=1.5733333333333333e-09}, {"Ic (+) (A)"=1.5733333333333329e-09, "Ic (-) (A)"=-1.5733333333333337e-09, "Ic (average) (A)"=1.5733333333333333e-09}, {"Ic (+) (A)"=7.466666666666674e-10, "Ic (-) (A)"=-1.1200000000000003e-09, "Ic (average) (A)"=9.333333333333338e-10}, {"Ic (+) (A)"=1.866666666666667e-09, "Ic (-) (A)"=-9.333333333333334e-10, "Ic (average) (A)"=1.4000000000000001e-09}, {"Ic (+) (A)"=1.4666666666666666e-09, "Ic (-) (A)"=-1.4133333333333334e-09, "Ic (average) (A)"=1.44e-09}, {"Ic (+) (A)"=8.266666666666671e-10, "Ic (-) (A)"=-2.453333333333333e-09, "Ic (average) (A)"=1.6400000000000001e-09}, {"Ic (+) (A)"=1.2266666666666674e-09, "Ic (-) (A)"=-7.2e-10, "Ic (average) (A)"=9.733333333333337e-10}, {"Ic (+) (A)"=3.466666666666671e-10, "Ic (-) (A)"=-1.8400000000000003e-09, "Ic (average) (A)"=1.0933333333333337e-09}, {"Ic (+) (A)"=1.626666666666666e-09, "Ic (-) (A)"=-7.733333333333331e-10, "Ic (average) (A)"=1.1999999999999996e-09}, {"Ic (+) (A)"=1.1199999999999994e-09, "Ic (-) (A)"=-1.2266666666666666e-09, "Ic (average) (A)"=1.173333333333333e-09}, {"Ic (+) (A)"=1.3333333333333337e-09, "Ic (-) (A)"=-7.733333333333331e-10, "Ic (average) (A)"=1.0533333333333334e-09}, {"Ic (+) (A)"=1.2800000000000005e-09, "Ic (-) (A)"=-8.800000000000003e-10, "Ic (average) (A)"=1.0800000000000004e-09}, {"Ic (+) (A)"=1.1733333333333326e-09, "Ic (-) (A)"=-1.5466666666666671e-09, "Ic (average) (A)"=1.3599999999999999e-09}, {"Ic (+) (A)"=0.0, "Ic (-) (A)"=-1.44e-09, "Ic (average) (A)"=7.2e-10}, {"Ic (+) (A)"=1.253333333333334e-09, "Ic (-) (A)"=-1.866666666666667e-09, "Ic (average) (A)"=1.5600000000000004e-09}, {"Ic (+) (A)"=1.0399999999999997e-09, "Ic (-) (A)"=-5.333333333333315e-11, "Ic (average) (A)"=5.466666666666664e-10}, {"Ic (+) (A)"=6.933333333333326e-10, "Ic (-) (A)"=-6.133333333333337e-10, "Ic (average) (A)"=6.533333333333331e-10}, {"Ic (+) (A)"=1.5199999999999997e-09, "Ic (-) (A)"=-4.8e-10, "Ic (average) (A)"=9.999999999999999e-10}, {"Ic (+) (A)"=9.333333333333334e-10, "Ic (-) (A)"=-1.5733333333333337e-09, "Ic (average) (A)"=1.2533333333333336e-09}, {"Ic (+) (A)"=4.533333333333334e-10, "Ic (-) (A)"=-1.68e-09, "Ic (average) (A)"=1.0666666666666667e-09}, {"Ic (+) (A)"=9.333333333333334e-10, "Ic (-) (A)"=-1.3600000000000003e-09, "Ic (average) (A)"=1.1466666666666668e-09}, {"Ic (+) (A)"=1.1733333333333326e-09, "Ic (-) (A)"=-3.466666666666671e-10, "Ic (average) (A)"=7.599999999999999e-10}, {"Ic (+) (A)"=1.3600000000000003e-09, "Ic (-) (A)"=-2.93333333333334e-10, "Ic (average) (A)"=8.266666666666671e-10}, {"Ic (+) (A)"=6.133333333333329e-10, "Ic (-) (A)"=-1.6533333333333334e-09, "Ic (average) (A)"=1.1333333333333331e-09}, {"Ic (+) (A)"=1.2000000000000008e-09, "Ic (-) (A)"=-5.866666666666671e-10, "Ic (average) (A)"=8.93333333333334e-10}, {"Ic (+) (A)"=5.333333333333315e-11, "Ic (-) (A)"=-1.4133333333333334e-09, "Ic (average) (A)"=7.333333333333333e-10}, {"Ic (+) (A)"=2.93333333333334e-10, "Ic (-) (A)"=-5.066666666666666e-10, "Ic (average) (A)"=4.0000000000000027e-10}, {"Ic (+) (A)"=1.3333333333333337e-09, "Ic (-) (A)"=-6.666666666666668e-10, "Ic (average) (A)"=1.0000000000000003e-09}, {"Ic (+) (A)"=1.146666666666666e-09, "Ic (-) (A)"=-3.733333333333337e-10, "Ic (average) (A)"=7.599999999999999e-10}, {"Ic (+) (A)"=1.0666666666666663e-09, "Ic (-) (A)"=-7.733333333333331e-10, "Ic (average) (A)"=9.199999999999997e-10}, {"Ic (+) (A)"=1.8666666666666602e-10, "Ic (-) (A)"=-6.666666666666668e-10, "Ic (average) (A)"=4.2666666666666643e-10}, {"Ic (+) (A)"=3.733333333333337e-10, "Ic (-) (A)"=-1.4666666666666666e-09, "Ic (average) (A)"=9.200000000000001e-10}, {"Ic (+) (A)"=3.2000000000000055e-10, "Ic (-) (A)"=-1.2799999999999997e-09, "Ic (average) (A)"=8.000000000000001e-10}, {"Ic (+) (A)"=3.2000000000000055e-10, "Ic (-) (A)"=-7.999999999999997e-10, "Ic (average) (A)"=5.600000000000001e-10}, {"Ic (+) (A)"=3.2000000000000055e-10, "Ic (-) (A)"=-2.133333333333326e-10, "Ic (average) (A)"=2.6666666666666657e-10}, {"Ic (+) (A)"=2.666666666666674e-10, "Ic (-) (A)"=-7.999999999999997e-10, "Ic (average) (A)"=5.333333333333336e-10}, {"Ic (+) (A)"=1.253333333333334e-09, "Ic (-) (A)"=-1.5999999999999945e-10, "Ic (average) (A)"=7.066666666666667e-10}, {"Ic (+) (A)"=4.533333333333334e-10, "Ic (-) (A)"=-1.066666666666663e-10, "Ic (average) (A)"=2.7999999999999986e-10}, {"Ic (+) (A)"=1.253333333333334e-09, "Ic (-) (A)"=-2.400000000000008e-10, "Ic (average) (A)"=7.466666666666674e-10}, {"Ic (+) (A)"=2.400000000000008e-10, "Ic (-) (A)"=-5.333333333333331e-10, "Ic (average) (A)"=3.86666666666667e-10}, {"Ic (+) (A)"=7.999999999999972e-11, "Ic (-) (A)"=-1.2799999999999997e-09, "Ic (average) (A)"=6.799999999999997e-10}, {"Ic (+) (A)"=1.2000000000000008e-09, "Ic (-) (A)"=-1.0666666666666671e-09, "Ic (average) (A)"=1.133333333333334e-09}, {"Ic (+) (A)"=6.399999999999994e-10, "Ic (-) (A)"=-7.999999999999997e-10, "Ic (average) (A)"=7.199999999999996e-10}, {"Ic (+) (A)"=2.666666666666674e-10, "Ic (-) (A)"=-3.466666666666671e-10, "Ic (average) (A)"=3.0666666666666726e-10}, {"Ic (+) (A)"=5.333333333333331e-10, "Ic (-) (A)"=-2.6666666666666575e-11, "Ic (average) (A)"=2.7999999999999986e-10}, {"Ic (+) (A)"=2.133333333333326e-10, "Ic (-) (A)"=-1.3333333333333287e-10, "Ic (average) (A)"=1.7333333333333273e-10}, {"Ic (+) (A)"=2.93333333333334e-10, "Ic (-) (A)"=-1.3333333333333287e-10, "Ic (average) (A)"=2.1333333333333342e-10}, {"Ic (+) (A)"=7.999999999999972e-11, "Ic (-) (A)"=-3.733333333333337e-10, "Ic (average) (A)"=2.266666666666667e-10}, {"Ic (+) (A)"=5.066666666666666e-10, "Ic (-) (A)"=-5.333333333333331e-10, "Ic (average) (A)"=5.199999999999999e-10}, {"Ic (+) (A)"=5.333333333333331e-10, "Ic (-) (A)"=-2.93333333333334e-10, "Ic (average) (A)"=4.1333333333333356e-10}, {"Ic (+) (A)"=6.399999999999994e-10, "Ic (-) (A)"=-2.400000000000008e-10, "Ic (average) (A)"=4.4000000000000013e-10}, {"Ic (+) (A)"=1.3333333333333287e-10, "Ic (-) (A)"=-1.066666666666663e-10, "Ic (average) (A)"=1.1999999999999959e-10}, {"Ic (+) (A)"=9.333333333333334e-10, "Ic (-) (A)"=-2.6666666666666575e-11, "Ic (average) (A)"=4.8e-10}, {"Ic (+) (A)"=8.266666666666671e-10, "Ic (-) (A)"=-1.066666666666663e-10, "Ic (average) (A)"=4.666666666666667e-10}, {"Ic (+) (A)"=9.066666666666668e-10, "Ic (-) (A)"=-1.8666666666666602e-10, "Ic (average) (A)"=5.466666666666664e-10}, {"Ic (+) (A)"=1.5999999999999945e-10, "Ic (-) (A)"=-2.93333333333334e-10, "Ic (average) (A)"=2.266666666666667e-10}, {"Ic (+) (A)"=1.3333333333333287e-10, "Ic (-) (A)"=-3.733333333333337e-10, "Ic (average) (A)"=2.533333333333333e-10}, {"Ic (+) (A)"=5.333333333333331e-10, "Ic (-) (A)"=-5.333333333333331e-10, "Ic (average) (A)"=5.333333333333331e-10}, {"Ic (+) (A)"=2.93333333333334e-10, "Ic (-) (A)"=-6.933333333333334e-10, "Ic (average) (A)"=4.933333333333337e-10}, {"Ic (+) (A)"=4.533333333333334e-10, "Ic (-) (A)"=-3.733333333333337e-10, "Ic (average) (A)"=4.1333333333333356e-10}, {"Ic (+) (A)"=2.400000000000008e-10, "Ic (-) (A)"=-6.666666666666668e-10, "Ic (average) (A)"=4.5333333333333384e-10}, {"Ic (+) (A)"=3.733333333333337e-10, "Ic (-) (A)"=-1.8666666666666602e-10, "Ic (average) (A)"=2.7999999999999986e-10}, {"Ic (+) (A)"=8.266666666666671e-10, "Ic (-) (A)"=-2.6666666666666575e-11, "Ic (average) (A)"=4.2666666666666685e-10}, {"Ic (+) (A)"=6.66666666666666e-10, "Ic (-) (A)"=-1.8666666666666602e-10, "Ic (average) (A)"=4.26666666666666e-10}, {"Ic (+) (A)"=2.6666666666666575e-11, "Ic (-) (A)"=-2.400000000000008e-10, "Ic (average) (A)"=1.333333333333337e-10}, {"Ic (+) (A)"=2.400000000000008e-10, "Ic (-) (A)"=-7.466666666666666e-10, "Ic (average) (A)"=4.933333333333337e-10}, {"Ic (+) (A)"=0.0, "Ic (-) (A)"=-5.066666666666666e-10, "Ic (average) (A)"=2.533333333333333e-10}, {"Ic (+) (A)"=5.066666666666666e-10, "Ic (-) (A)"=-2.666666666666674e-10, "Ic (average) (A)"=3.86666666666667e-10}, {"Ic (+) (A)"=7.73333333333334e-10, "Ic (-) (A)"=-6.933333333333334e-10, "Ic (average) (A)"=7.333333333333337e-10}, {"Ic (+) (A)"=6.66666666666666e-10, "Ic (-) (A)"=-2.133333333333326e-10, "Ic (average) (A)"=4.399999999999993e-10}, {"Ic (+) (A)"=2.6666666666666575e-11, "Ic (-) (A)"=-1.0933333333333337e-09, "Ic (average) (A)"=5.600000000000001e-10}, {"Ic (+) (A)"=1.5999999999999945e-10, "Ic (-) (A)"=-5.599999999999997e-10, "Ic (average) (A)"=3.599999999999996e-10}, {"Ic (+) (A)"=1.066666666666663e-10, "Ic (-) (A)"=-2.400000000000008e-10, "Ic (average) (A)"=1.7333333333333356e-10}, {"Ic (+) (A)"=3.733333333333337e-10, "Ic (-) (A)"=-3.466666666666671e-10, "Ic (average) (A)"=3.600000000000004e-10}, {"Ic (+) (A)"=7.200000000000008e-10, "Ic (-) (A)"=-1.066666666666663e-10, "Ic (average) (A)"=4.1333333333333356e-10}, {"Ic (+) (A)"=5.333333333333315e-11, "Ic (-) (A)"=-4.533333333333334e-10, "Ic (average) (A)"=2.533333333333333e-10}, {"Ic (+) (A)"=2.666666666666674e-10, "Ic (-) (A)"=-1.3333333333333287e-10, "Ic (average) (A)"=2.0000000000000014e-10}, {"Ic (+) (A)"=9.333333333333334e-10, "Ic (-) (A)"=-7.999999999999972e-11, "Ic (average) (A)"=5.066666666666666e-10}, {"Ic (+) (A)"=5.066666666666666e-10, "Ic (-) (A)"=-5.333333333333315e-11, "Ic (average) (A)"=2.7999999999999986e-10}, {"Ic (+) (A)"=1.066666666666663e-10, "Ic (-) (A)"=-5.599999999999997e-10, "Ic (average) (A)"=3.33333333333333e-10}, {"Ic (+) (A)"=4.0000000000000027e-10, "Ic (-) (A)"=-7.999999999999997e-10, "Ic (average) (A)"=6e-10}, {"Ic (+) (A)"=3.466666666666671e-10, "Ic (-) (A)"=-1.066666666666663e-10, "Ic (average) (A)"=2.266666666666667e-10}, {"Ic (+) (A)"=7.200000000000008e-10, "Ic (-) (A)"=-4.0000000000000027e-10, "Ic (average) (A)"=5.600000000000005e-10}, {"Ic (+) (A)"=7.200000000000008e-10, "Ic (-) (A)"=-2.6666666666666575e-11, "Ic (average) (A)"=3.733333333333337e-10}, {"Ic (+) (A)"=4.0000000000000027e-10, "Ic (-) (A)"=-1.3333333333333287e-10, "Ic (average) (A)"=2.6666666666666657e-10}, {"Ic (+) (A)"=7.999999999999972e-11, "Ic (-) (A)"=-7.999999999999997e-10, "Ic (average) (A)"=4.399999999999997e-10}, {"Ic (+) (A)"=8.000000000000005e-10, "Ic (-) (A)"=-7.999999999999972e-11, "Ic (average) (A)"=4.4000000000000013e-10}, {"Ic (+) (A)"=4.2666666666666685e-10, "Ic (-) (A)"=-1.066666666666663e-10, "Ic (average) (A)"=2.6666666666666657e-10}, {"Ic (+) (A)"=5.066666666666666e-10, "Ic (-) (A)"=-9.6e-10, "Ic (average) (A)"=7.333333333333333e-10}, {"Ic (+) (A)"=0.0, "Ic (-) (A)"=-8.266666666666671e-10, "Ic (average) (A)"=4.1333333333333356e-10}, {"Ic (+) (A)"=3.2000000000000055e-10, "Ic (-) (A)"=-2.133333333333326e-10, "Ic (average) (A)"=2.6666666666666657e-10}, {"Ic (+) (A)"=1.5999999999999945e-10, "Ic (-) (A)"=-1.3600000000000003e-09, "Ic (average) (A)"=7.599999999999999e-10}, {"Ic (+) (A)"=5.333333333333315e-11, "Ic (-) (A)"=-2.6666666666666575e-11, "Ic (average) (A)"=3.999999999999986e-11}, {"Ic (+) (A)"=1.066666666666663e-10, "Ic (-) (A)"=-4.533333333333334e-10, "Ic (average) (A)"=2.7999999999999986e-10}, {"Ic (+) (A)"=4.8e-10, "Ic (-) (A)"=-1.8666666666666602e-10, "Ic (average) (A)"=3.33333333333333e-10}, {"Ic (+) (A)"=0.0, "Ic (-) (A)"=-1.0133333333333331e-09, "Ic (average) (A)"=5.066666666666666e-10}, {"Ic (+) (A)"=9.066666666666668e-10, "Ic (-) (A)"=-2.133333333333326e-10, "Ic (average) (A)"=5.599999999999997e-10}, {"Ic (+) (A)"=1.066666666666663e-10, "Ic (-) (A)"=-2.133333333333326e-10, "Ic (average) (A)"=1.5999999999999945e-10}, {"Ic (+) (A)"=1.066666666666663e-10, "Ic (-) (A)"=-2.666666666666674e-10, "Ic (average) (A)"=1.8666666666666685e-10}, {"Ic (+) (A)"=1.8666666666666602e-10, "Ic (-) (A)"=-2.666666666666674e-10, "Ic (average) (A)"=2.266666666666667e-10}, {"Ic (+) (A)"=5.599999999999997e-10, "Ic (-) (A)"=-4.0000000000000027e-10, "Ic (average) (A)"=4.8e-10}, {"Ic (+) (A)"=9.066666666666668e-10, "Ic (-) (A)"=-2.400000000000008e-10, "Ic (average) (A)"=5.733333333333338e-10}, {"Ic (+) (A)"=6.399999999999994e-10, "Ic (-) (A)"=-2.93333333333334e-10, "Ic (average) (A)"=4.666666666666667e-10}, {"Ic (+) (A)"=2.6666666666666575e-11, "Ic (-) (A)"=-3.2000000000000055e-10, "Ic (average) (A)"=1.7333333333333356e-10}, {"Ic (+) (A)"=2.93333333333334e-10, "Ic (-) (A)"=-2.666666666666674e-10, "Ic (average) (A)"=2.800000000000007e-10}, {"Ic (+) (A)"=2.133333333333326e-10, "Ic (-) (A)"=-2.6666666666666575e-11, "Ic (average) (A)"=1.1999999999999959e-10}, {"Ic (+) (A)"=5.066666666666666e-10, "Ic (-) (A)"=-1.8666666666666602e-10, "Ic (average) (A)"=3.466666666666663e-10}, {"Ic (+) (A)"=6.933333333333326e-10, "Ic (-) (A)"=-2.400000000000008e-10, "Ic (average) (A)"=4.666666666666667e-10}, {"Ic (+) (A)"=5.333333333333315e-11, "Ic (-) (A)"=-3.466666666666671e-10, "Ic (average) (A)"=2.0000000000000014e-10}, {"Ic (+) (A)"=2.93333333333334e-10, "Ic (-) (A)"=-1.0933333333333337e-09, "Ic (average) (A)"=6.933333333333338e-10}, {"Ic (+) (A)"=5.599999999999997e-10, "Ic (-) (A)"=-1.5999999999999945e-10, "Ic (average) (A)"=3.599999999999996e-10}, {"Ic (+) (A)"=5.333333333333315e-11, "Ic (-) (A)"=-7.733333333333331e-10, "Ic (average) (A)"=4.1333333333333315e-10}, {"Ic (+) (A)"=2.6666666666666575e-11, "Ic (-) (A)"=-2.400000000000008e-10, "Ic (average) (A)"=1.333333333333337e-10}, {"Ic (+) (A)"=1.066666666666663e-10, "Ic (-) (A)"=-2.133333333333326e-10, "Ic (average) (A)"=1.5999999999999945e-10}, {"Ic (+) (A)"=7.999999999999972e-11, "Ic (-) (A)"=-4.0000000000000027e-10, "Ic (average) (A)"=2.4e-10}, {"Ic (+) (A)"=7.999999999999972e-11, "Ic (-) (A)"=-2.666666666666674e-10, "Ic (average) (A)"=1.7333333333333356e-10}, {"Ic (+) (A)"=1.8666666666666602e-10, "Ic (-) (A)"=-5.333333333333315e-11, "Ic (average) (A)"=1.1999999999999959e-10}, {"Ic (+) (A)"=7.999999999999972e-11, "Ic (-) (A)"=-4.8e-10, "Ic (average) (A)"=2.7999999999999986e-10}, {"Ic (+) (A)"=5.599999999999997e-10, "Ic (-) (A)"=-4.0000000000000027e-10, "Ic (average) (A)"=4.8e-10}, {"Ic (+) (A)"=2.666666666666674e-10, "Ic (-) (A)"=-8.266666666666671e-10, "Ic (average) (A)"=5.466666666666673e-10}, {"Ic (+) (A)"=3.733333333333337e-10, "Ic (-) (A)"=-6.666666666666668e-10, "Ic (average) (A)"=5.200000000000003e-10}, {"Ic (+) (A)"=7.999999999999972e-11, "Ic (-) (A)"=-4.0000000000000027e-10, "Ic (average) (A)"=2.4e-10}, {"Ic (+) (A)"=2.400000000000008e-10, "Ic (-) (A)"=-6.133333333333337e-10, "Ic (average) (A)"=4.2666666666666726e-10}, {"Ic (+) (A)"=1.2800000000000005e-09, "Ic (-) (A)"=-1.1733333333333334e-09, "Ic (average) (A)"=1.226666666666667e-09}, {"Ic (+) (A)"=0.0, "Ic (-) (A)"=-5.333333333333331e-10, "Ic (average) (A)"=2.6666666666666657e-10}, {"Ic (+) (A)"=4.533333333333334e-10, "Ic (-) (A)"=-7.999999999999997e-10, "Ic (average) (A)"=6.266666666666666e-10}, {"Ic (+) (A)"=1.5999999999999945e-10, "Ic (-) (A)"=-7.733333333333331e-10, "Ic (average) (A)"=4.666666666666663e-10}, {"Ic (+) (A)"=1.1733333333333326e-09, "Ic (-) (A)"=-3.466666666666671e-10, "Ic (average) (A)"=7.599999999999999e-10}, {"Ic (+) (A)"=7.466666666666674e-10, "Ic (-) (A)"=-1.4133333333333334e-09, "Ic (average) (A)"=1.0800000000000004e-09}, {"Ic (+) (A)"=1.066666666666663e-10, "Ic (-) (A)"=-6.666666666666668e-10, "Ic (average) (A)"=3.8666666666666657e-10}, {"Ic (+) (A)"=1.253333333333334e-09, "Ic (-) (A)"=-1.2e-09, "Ic (average) (A)"=1.226666666666667e-09}, {"Ic (+) (A)"=4.8e-10, "Ic (-) (A)"=-1.68e-09, "Ic (average) (A)"=1.08e-09}, {"Ic (+) (A)"=9.6e-10, "Ic (-) (A)"=-1.0933333333333337e-09, "Ic (average) (A)"=1.0266666666666668e-09}, {"Ic (+) (A)"=1.4666666666666666e-09, "Ic (-) (A)"=-1.2266666666666666e-09, "Ic (average) (A)"=1.3466666666666666e-09}, {"Ic (+) (A)"=1.146666666666666e-09, "Ic (-) (A)"=-1.0399999999999997e-09, "Ic (average) (A)"=1.0933333333333329e-09}, {"Ic (+) (A)"=1.2266666666666674e-09, "Ic (-) (A)"=-1.6533333333333334e-09, "Ic (average) (A)"=1.4400000000000004e-09}, {"Ic (+) (A)"=1.3600000000000003e-09, "Ic (-) (A)"=-1.0133333333333331e-09, "Ic (average) (A)"=1.1866666666666667e-09}, {"Ic (+) (A)"=1.3866666666666668e-09, "Ic (-) (A)"=-1.7333333333333331e-09, "Ic (average) (A)"=1.56e-09}, {"Ic (+) (A)"=1.5466666666666663e-09, "Ic (-) (A)"=-6.666666666666668e-10, "Ic (average) (A)"=1.1066666666666666e-09}, {"Ic (+) (A)"=1.5199999999999997e-09, "Ic (-) (A)"=-2.346666666666667e-09, "Ic (average) (A)"=1.9333333333333333e-09}, {"Ic (+) (A)"=1.3066666666666671e-09, "Ic (-) (A)"=-1.0933333333333337e-09, "Ic (average) (A)"=1.2000000000000004e-09}, {"Ic (+) (A)"=1.2000000000000008e-09, "Ic (-) (A)"=-1.8133333333333337e-09, "Ic (average) (A)"=1.5066666666666673e-09}, {"Ic (+) (A)"=1.7066666666666674e-09, "Ic (-) (A)"=-1.3866666666666668e-09, "Ic (average) (A)"=1.5466666666666671e-09}, {"Ic (+) (A)"=1.0399999999999997e-09, "Ic (-) (A)"=-1.4666666666666666e-09, "Ic (average) (A)"=1.2533333333333331e-09}, {"Ic (+) (A)"=1.866666666666667e-09, "Ic (-) (A)"=-2.1333333333333334e-09, "Ic (average) (A)"=2e-09}, {"Ic (+) (A)"=1.8133333333333337e-09, "Ic (-) (A)"=-1.5199999999999997e-09, "Ic (average) (A)"=1.6666666666666667e-09}, {"Ic (+) (A)"=2.0799999999999994e-09, "Ic (-) (A)"=-1.7066666666666666e-09, "Ic (average) (A)"=1.893333333333333e-09}, {"Ic (+) (A)"=1.973333333333333e-09, "Ic (-) (A)"=-2.0800000000000003e-09, "Ic (average) (A)"=2.0266666666666667e-09}, {"Ic (+) (A)"=1.92e-09, "Ic (-) (A)"=-1.2799999999999997e-09, "Ic (average) (A)"=1.5999999999999999e-09}, {"Ic (+) (A)"=3.0399999999999994e-09, "Ic (-) (A)"=-2.026666666666667e-09, "Ic (average) (A)"=2.5333333333333333e-09}, {"Ic (+) (A)"=1.7600000000000005e-09, "Ic (-) (A)"=-2.1866666666666666e-09, "Ic (average) (A)"=1.9733333333333335e-09}, {"Ic (+) (A)"=2.640000000000001e-09, "Ic (-) (A)"=-2.1866666666666666e-09, "Ic (average) (A)"=2.4133333333333337e-09}, {"Ic (+) (A)"=1.973333333333333e-09, "Ic (-) (A)"=-2.213333333333333e-09, "Ic (average) (A)"=2.093333333333333e-09}, {"Ic (+) (A)"=2.0266666666666663e-09, "Ic (-) (A)"=-2.3733333333333334e-09, "Ic (average) (A)"=2.2e-09}, {"Ic (+) (A)"=2.0799999999999994e-09, "Ic (-) (A)"=-2.3200000000000003e-09, "Ic (average) (A)"=2.2e-09}, {"Ic (+) (A)"=2.1866666666666674e-09, "Ic (-) (A)"=-2.3200000000000003e-09, "Ic (average) (A)"=2.253333333333334e-09}, {"Ic (+) (A)"=2.2933333333333337e-09, "Ic (-) (A)"=-2.2400000000000005e-09, "Ic (average) (A)"=2.266666666666667e-09}, {"Ic (+) (A)"=2.0799999999999994e-09, "Ic (-) (A)"=-2.3733333333333334e-09, "Ic (average) (A)"=2.2266666666666664e-09}, {"Ic (+) (A)"=2.160000000000001e-09, "Ic (-) (A)"=-2.346666666666667e-09, "Ic (average) (A)"=2.253333333333334e-09}, {"Ic (+) (A)"=2.266666666666667e-09, "Ic (-) (A)"=-2.3733333333333334e-09, "Ic (average) (A)"=2.3200000000000003e-09}, {"Ic (+) (A)"=2.346666666666667e-09, "Ic (-) (A)"=-2.4800000000000005e-09, "Ic (average) (A)"=2.4133333333333337e-09}, {"Ic (+) (A)"=2.7733333333333337e-09, "Ic (-) (A)"=-2.5333333333333337e-09, "Ic (average) (A)"=2.6533333333333337e-09}, {"Ic (+) (A)"=2.2933333333333337e-09, "Ic (-) (A)"=-2.4800000000000005e-09, "Ic (average) (A)"=2.386666666666667e-09}, {"Ic (+) (A)"=2.346666666666667e-09, "Ic (-) (A)"=-2.5600000000000003e-09, "Ic (average) (A)"=2.4533333333333335e-09}, {"Ic (+) (A)"=2.4e-09, "Ic (-) (A)"=-2.4800000000000005e-09, "Ic (average) (A)"=2.4400000000000003e-09}, {"Ic (+) (A)"=2.4799999999999997e-09, "Ic (-) (A)"=-2.7200000000000005e-09, "Ic (average) (A)"=2.6e-09}, {"Ic (+) (A)"=2.5066666666666663e-09, "Ic (-) (A)"=-2.693333333333333e-09, "Ic (average) (A)"=2.5999999999999997e-09}, {"Ic (+) (A)"=2.5066666666666663e-09, "Ic (-) (A)"=-2.746666666666667e-09, "Ic (average) (A)"=2.6266666666666667e-09}, {"Ic (+) (A)"=2.533333333333333e-09, "Ic (-) (A)"=-2.4800000000000005e-09, "Ic (average) (A)"=2.5066666666666667e-09}, {"Ic (+) (A)"=2.693333333333334e-09, "Ic (-) (A)"=-2.9066666666666666e-09, "Ic (average) (A)"=2.8000000000000003e-09}, {"Ic (+) (A)"=2.746666666666667e-09, "Ic (-) (A)"=-2.933333333333333e-09, "Ic (average) (A)"=2.84e-09}, {"Ic (+) (A)"=2.826666666666667e-09, "Ic (-) (A)"=-2.8000000000000003e-09, "Ic (average) (A)"=2.8133333333333335e-09}, {"Ic (+) (A)"=3.0399999999999994e-09, "Ic (-) (A)"=-2.8533333333333334e-09, "Ic (average) (A)"=2.9466666666666664e-09}, {"Ic (+) (A)"=2.933333333333333e-09, "Ic (-) (A)"=-3.2800000000000003e-09, "Ic (average) (A)"=3.1066666666666667e-09}, {"Ic (+) (A)"=2.8533333333333334e-09, "Ic (-) (A)"=-3.0933333333333334e-09, "Ic (average) (A)"=2.9733333333333334e-09}, {"Ic (+) (A)"=2.8000000000000003e-09, "Ic (-) (A)"=-3.0400000000000003e-09, "Ic (average) (A)"=2.9200000000000003e-09}, {"Ic (+) (A)"=2.8000000000000003e-09, "Ic (-) (A)"=-2.986666666666667e-09, "Ic (average) (A)"=2.8933333333333337e-09}, {"Ic (+) (A)"=2.9599999999999997e-09, "Ic (-) (A)"=-2.9600000000000005e-09, "Ic (average) (A)"=2.96e-09}, {"Ic (+) (A)"=2.88e-09, "Ic (-) (A)"=-3.1466666666666666e-09, "Ic (average) (A)"=3.0133333333333333e-09}, {"Ic (+) (A)"=2.9599999999999997e-09, "Ic (-) (A)"=-3.0933333333333334e-09, "Ic (average) (A)"=3.0266666666666666e-09}, {"Ic (+) (A)"=2.9599999999999997e-09, "Ic (-) (A)"=-2.933333333333333e-09, "Ic (average) (A)"=2.9466666666666664e-09}, {"Ic (+) (A)"=3.0666666666666677e-09, "Ic (-) (A)"=-3.2533333333333337e-09, "Ic (average) (A)"=3.1600000000000007e-09}, {"Ic (+) (A)"=3.0933333333333342e-09, "Ic (-) (A)"=-3.2533333333333337e-09, "Ic (average) (A)"=3.173333333333334e-09}, {"Ic (+) (A)"=3.0399999999999994e-09, "Ic (-) (A)"=-3.2533333333333337e-09, "Ic (average) (A)"=3.1466666666666666e-09}, {"Ic (+) (A)"=3.173333333333334e-09, "Ic (-) (A)"=-3.3866666666666666e-09, "Ic (average) (A)"=3.2800000000000003e-09}, {"Ic (+) (A)"=3.120000000000001e-09, "Ic (-) (A)"=-3.36e-09, "Ic (average) (A)"=3.2400000000000004e-09}, {"Ic (+) (A)"=3.120000000000001e-09, "Ic (-) (A)"=-3.306666666666667e-09, "Ic (average) (A)"=3.213333333333334e-09}, {"Ic (+) (A)"=3.226666666666667e-09, "Ic (-) (A)"=-3.466666666666667e-09, "Ic (average) (A)"=3.346666666666667e-09}, {"Ic (+) (A)"=3.306666666666667e-09, "Ic (-) (A)"=-3.4933333333333337e-09, "Ic (average) (A)"=3.4000000000000003e-09}, {"Ic (+) (A)"=3.3333333333333334e-09, "Ic (-) (A)"=-3.6800000000000005e-09, "Ic (average) (A)"=3.506666666666667e-09}, {"Ic (+) (A)"=3.413333333333333e-09, "Ic (-) (A)"=-3.6800000000000005e-09, "Ic (average) (A)"=3.546666666666667e-09}, {"Ic (+) (A)"=3.4399999999999997e-09, "Ic (-) (A)"=-3.5733333333333334e-09, "Ic (average) (A)"=3.5066666666666666e-09}, {"Ic (+) (A)"=3.5199999999999994e-09, "Ic (-) (A)"=-3.6266666666666666e-09, "Ic (average) (A)"=3.573333333333333e-09}, {"Ic (+) (A)"=3.4399999999999997e-09, "Ic (-) (A)"=-3.733333333333334e-09, "Ic (average) (A)"=3.5866666666666667e-09}, {"Ic (+) (A)"=3.493333333333333e-09, "Ic (-) (A)"=-3.5733333333333334e-09, "Ic (average) (A)"=3.533333333333333e-09}, {"Ic (+) (A)"=3.5199999999999994e-09, "Ic (-) (A)"=-3.813333333333333e-09, "Ic (average) (A)"=3.6666666666666664e-09}, {"Ic (+) (A)"=3.893333333333333e-09, "Ic (-) (A)"=-3.786666666666667e-09, "Ic (average) (A)"=3.84e-09}, {"Ic (+) (A)"=3.8666666666666665e-09, "Ic (-) (A)"=-3.76e-09, "Ic (average) (A)"=3.813333333333333e-09}, {"Ic (+) (A)"=3.5733333333333342e-09, "Ic (-) (A)"=-3.76e-09, "Ic (average) (A)"=3.6666666666666672e-09}, {"Ic (+) (A)"=3.600000000000001e-09, "Ic (-) (A)"=-3.76e-09, "Ic (average) (A)"=3.6800000000000005e-09}, {"Ic (+) (A)"=3.600000000000001e-09, "Ic (-) (A)"=-3.706666666666667e-09, "Ic (average) (A)"=3.653333333333334e-09}, {"Ic (+) (A)"=3.600000000000001e-09, "Ic (-) (A)"=-3.813333333333333e-09, "Ic (average) (A)"=3.706666666666667e-09}, {"Ic (+) (A)"=3.6800000000000005e-09, "Ic (-) (A)"=-4.453333333333334e-09, "Ic (average) (A)"=4.066666666666667e-09}, {"Ic (+) (A)"=3.733333333333334e-09, "Ic (-) (A)"=-3.9200000000000005e-09, "Ic (average) (A)"=3.8266666666666675e-09}, {"Ic (+) (A)"=4.053333333333334e-09, "Ic (-) (A)"=-3.9200000000000005e-09, "Ic (average) (A)"=3.986666666666667e-09}, {"Ic (+) (A)"=3.84e-09, "Ic (-) (A)"=-4.053333333333333e-09, "Ic (average) (A)"=3.946666666666666e-09}, {"Ic (+) (A)"=3.786666666666667e-09, "Ic (-) (A)"=-4.053333333333333e-09, "Ic (average) (A)"=3.92e-09}, {"Ic (+) (A)"=3.893333333333333e-09, "Ic (-) (A)"=-4.1066666666666665e-09, "Ic (average) (A)"=3.9999999999999994e-09}, {"Ic (+) (A)"=3.92e-09, "Ic (-) (A)"=-4.186666666666667e-09, "Ic (average) (A)"=4.053333333333333e-09}, {"Ic (+) (A)"=3.973333333333333e-09, "Ic (-) (A)"=-4.266666666666667e-09, "Ic (average) (A)"=4.12e-09}, {"Ic (+) (A)"=3.973333333333333e-09, "Ic (-) (A)"=-4.186666666666667e-09, "Ic (average) (A)"=4.08e-09}, {"Ic (+) (A)"=4.080000000000001e-09, "Ic (-) (A)"=-4.4e-09, "Ic (average) (A)"=4.24e-09}, {"Ic (+) (A)"=4.053333333333334e-09, "Ic (-) (A)"=-4.293333333333333e-09, "Ic (average) (A)"=4.173333333333334e-09}, {"Ic (+) (A)"=4.1600000000000005e-09, "Ic (-) (A)"=-4.293333333333333e-09, "Ic (average) (A)"=4.226666666666667e-09}, {"Ic (+) (A)"=4.053333333333334e-09, "Ic (-) (A)"=-4.4e-09, "Ic (average) (A)"=4.226666666666667e-09}, {"Ic (+) (A)"=4.106666666666667e-09, "Ic (-) (A)"=-4.3466666666666665e-09, "Ic (average) (A)"=4.226666666666667e-09}, {"Ic (+) (A)"=4.1600000000000005e-09, "Ic (-) (A)"=-4.506666666666667e-09, "Ic (average) (A)"=4.333333333333334e-09}, {"Ic (+) (A)"=4.32e-09, "Ic (-) (A)"=-4.506666666666667e-09, "Ic (average) (A)"=4.413333333333334e-09}, {"Ic (+) (A)"=4.32e-09, "Ic (-) (A)"=-4.453333333333334e-09, "Ic (average) (A)"=4.386666666666667e-09}, {"Ic (+) (A)"=4.3466666666666665e-09, "Ic (-) (A)"=-4.560000000000001e-09, "Ic (average) (A)"=4.453333333333334e-09}, {"Ic (+) (A)"=4.453333333333333e-09, "Ic (-) (A)"=-4.586666666666667e-09, "Ic (average) (A)"=4.52e-09}, {"Ic (+) (A)"=4.480000000000001e-09, "Ic (-) (A)"=-4.560000000000001e-09, "Ic (average) (A)"=4.520000000000001e-09}, {"Ic (+) (A)"=4.453333333333333e-09, "Ic (-) (A)"=-4.6400000000000005e-09, "Ic (average) (A)"=4.546666666666667e-09}, {"Ic (+) (A)"=4.480000000000001e-09, "Ic (-) (A)"=-4.666666666666667e-09, "Ic (average) (A)"=4.573333333333334e-09}, {"Ic (+) (A)"=4.560000000000001e-09, "Ic (-) (A)"=-4.693333333333334e-09, "Ic (average) (A)"=4.626666666666667e-09}, {"Ic (+) (A)"=4.586666666666667e-09, "Ic (-) (A)"=-4.746666666666667e-09, "Ic (average) (A)"=4.666666666666667e-09}, {"Ic (+) (A)"=4.533333333333334e-09, "Ic (-) (A)"=-4.773333333333333e-09, "Ic (average) (A)"=4.653333333333334e-09}, {"Ic (+) (A)"=4.560000000000001e-09, "Ic (-) (A)"=-4.773333333333333e-09, "Ic (average) (A)"=4.666666666666667e-09}, {"Ic (+) (A)"=4.613333333333334e-09, "Ic (-) (A)"=-4.906666666666667e-09, "Ic (average) (A)"=4.760000000000001e-09}, {"Ic (+) (A)"=4.693333333333334e-09, "Ic (-) (A)"=-4.88e-09, "Ic (average) (A)"=4.786666666666667e-09}, {"Ic (+) (A)"=4.6400000000000005e-09, "Ic (-) (A)"=-4.933333333333334e-09, "Ic (average) (A)"=4.7866666666666675e-09}, {"Ic (+) (A)"=4.773333333333333e-09, "Ic (-) (A)"=-4.906666666666667e-09, "Ic (average) (A)"=4.840000000000001e-09}, {"Ic (+) (A)"=4.773333333333333e-09, "Ic (-) (A)"=-4.986666666666667e-09, "Ic (average) (A)"=4.88e-09}, {"Ic (+) (A)"=4.666666666666667e-09, "Ic (-) (A)"=-4.933333333333334e-09, "Ic (average) (A)"=4.8e-09}, {"Ic (+) (A)"=4.8e-09, "Ic (-) (A)"=-5.040000000000001e-09, "Ic (average) (A)"=4.92e-09}, {"Ic (+) (A)"=4.773333333333333e-09, "Ic (-) (A)"=-5.013333333333334e-09, "Ic (average) (A)"=4.893333333333334e-09}, {"Ic (+) (A)"=4.906666666666666e-09, "Ic (-) (A)"=-5.1200000000000005e-09, "Ic (average) (A)"=5.013333333333333e-09}, {"Ic (+) (A)"=4.906666666666666e-09, "Ic (-) (A)"=-5.066666666666667e-09, "Ic (average) (A)"=4.986666666666667e-09}, {"Ic (+) (A)"=4.906666666666666e-09, "Ic (-) (A)"=-5.173333333333334e-09, "Ic (average) (A)"=5.04e-09}, {"Ic (+) (A)"=4.933333333333333e-09, "Ic (-) (A)"=-5.1200000000000005e-09, "Ic (average) (A)"=5.026666666666667e-09}]
  out "Rc v Rn 2":cluster{i32[], dbl[]}[](graph)
  out "Rc v Rn":cluster{dbl[], dbl[]}(graph)
  in  "divider 2":dbl=1.0
  in  "N/SC fitting points":T2={"N-State Points to fit"=300.0, "SC-State Points to fit"=75.0, "Additional SC Center offset"=0.0}
  in  "Independent variable":string(combo)="Backgate Voltage (V)"
  in  "Tab Control":enum32{"IcRn", "Ic", "dV/dI vs Gate"}(tab)
  in  "Gate Voltages 1":dbl[](array[numeric])
  out "IcRn":cluster{i32[], dbl[]}(graph)
  in  "Input curves 2":cluster{dbl[], dbl[]}[](array[cluster])
  out "IcRn vs Rn":cluster{dbl[], dbl[]}(graph)
  in  "divider":dbl=8.51947e-09
  out "Ic":cluster{i32[], dbl[]}(graph)
  out "A vs B 4":dbl[][](graph)
  out "A vs B 3":cluster{dbl[], dbl[]}[](graph)
  in  "How many V sweep periods?":dbl=1.0
  in  "dV/dI (Ic) Parameters":T3={"High current value"=8e-09, "Low currentvalue"=-8e-09, "decimation points"=600, "side points"=8, "polynomial order 2"=4, "peak width"=18, "peak threshold"=50000.0, "trough threshold"=20000.0}
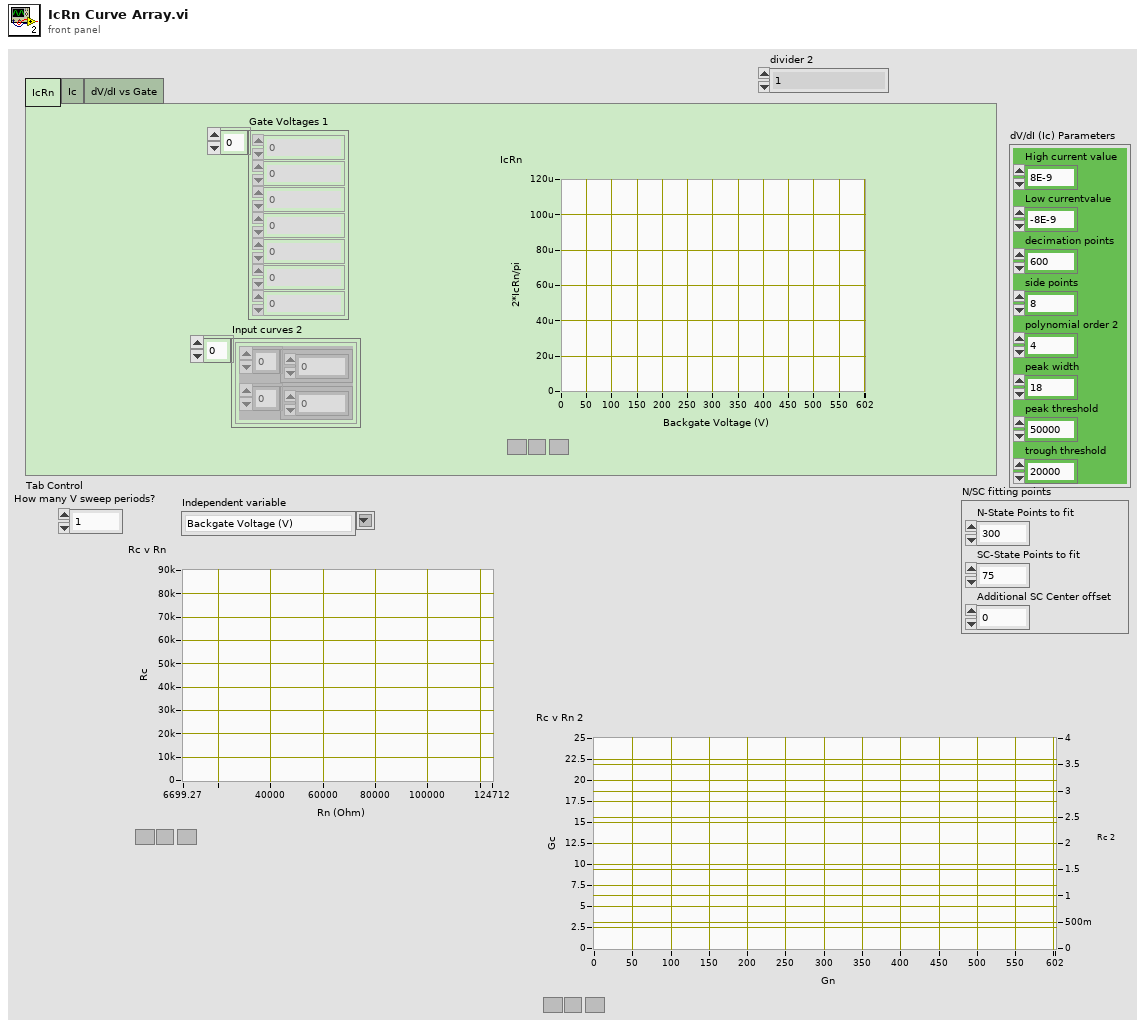
[diagram p1: front panel]
types:
  T1 = cluster{"Ic (+) (A)":dbl, "Ic (-) (A)":dbl, "Ic (average) (A)":dbl}[]
  T2 = cluster{"N-State Points to fit":dbl, "SC-State Points to fit":dbl, "Additional SC Center offset":dbl}
  T3 = cluster{"High current value":dbl, "Low currentvalue":dbl, "decimation points":i32, "side points":i32, "polynomial order 2":i32, "peak width":i32, "peak threshold":dbl, "trough threshold":dbl}
  T4 = cluster{"Ic (+) (A)":dbl, "Ic (-) (A)":dbl, "Ic (average) (A)":dbl}
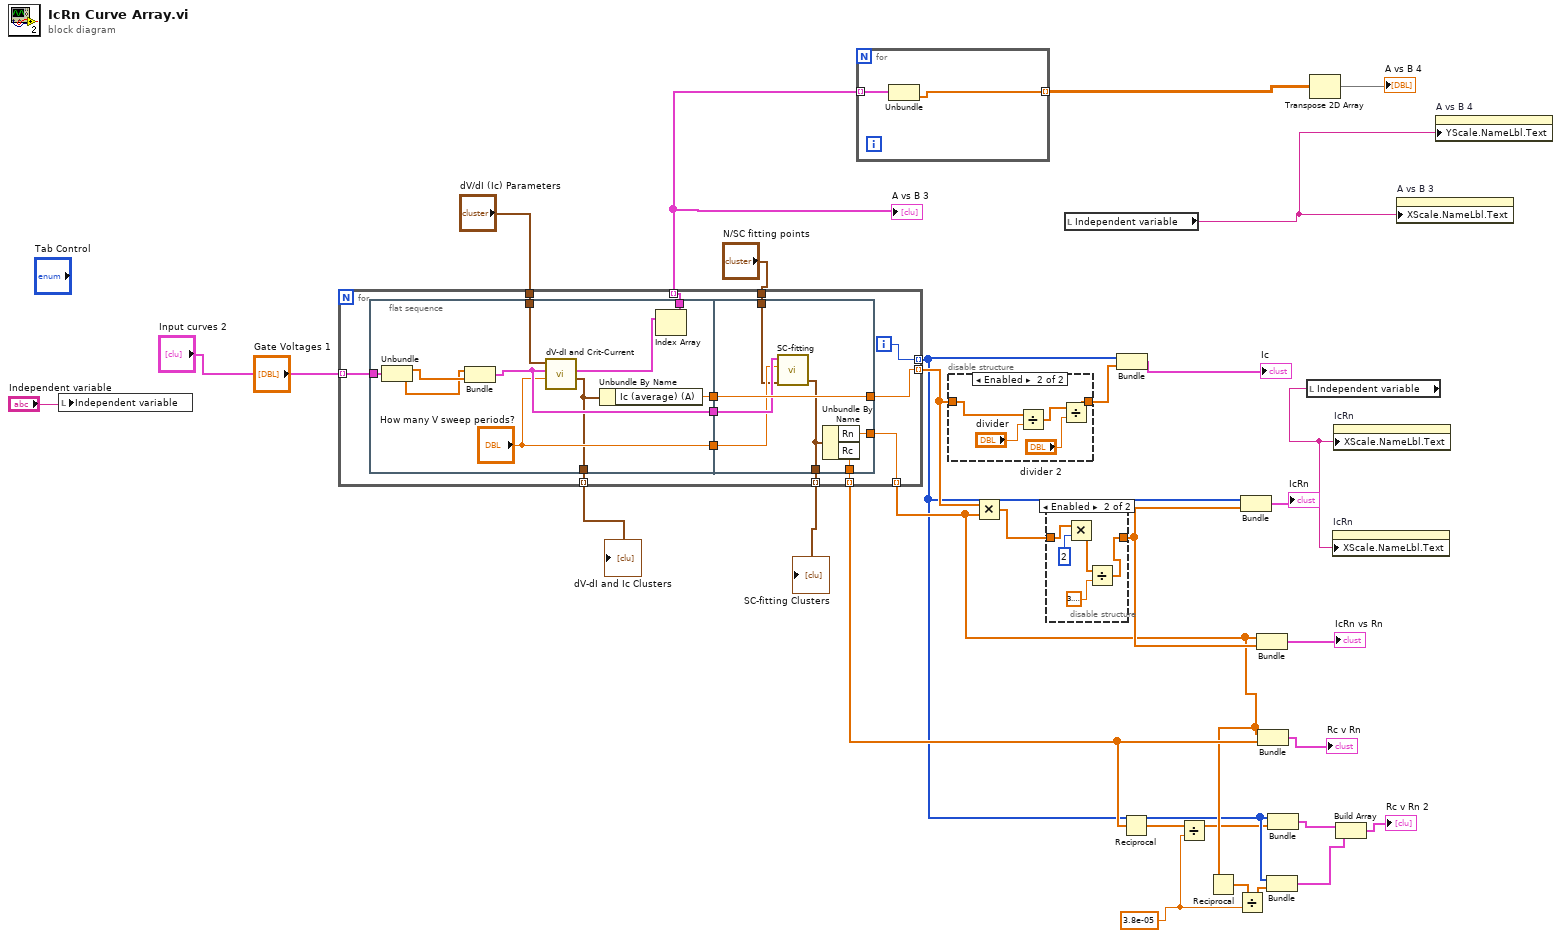
[diagram p0: block diagram]
diagram:
  w4 = 3.8e-05
  n1 = local write "Independent variable"("Independent variable") -> ()
  n2 = for {
    tunnel: "Input curves 2" -> [w42] mode=indexing
    tunnel: "dV/dI (Ic) Parameters" -> [w43]
    tunnel: [w41] -> w30 mode=indexing
    tunnel: [w40] -> w12 mode=indexing
    tunnel: [w39] -> w17 mode=indexing
    tunnel: "N/SC fitting points" -> [w35]
    tunnel: [w34] -> w13 mode=indexing
    tunnel: [w33] -> w14 mode=indexing
    tunnel: [w32] -> w3 mode=indexing
    tunnel: [w31] -> w2 mode=indexing
    i -> [w40]
    n3 = flat-sequence {
      tunnel: w43 -> [w53]
      tunnel: w42 -> [w52]
      tunnel: [w49] -> w41
      tunnel: [w47] -> w38
      tunnel: [w46] -> w37
      tunnel: ["How many V sweep periods?"] -> w36
      tunnel: [w44] -> w32
      tunnel: [w60] -> w39
      tunnel: w38 -> [w60]
      tunnel: w37 -> [w59]
      tunnel: w36 -> [w58]
      tunnel: w35 -> [w57]
      tunnel: [w56] -> w34
      tunnel: [w55] -> w33
      tunnel: [w54] -> w31
      frame #0 {
        n4 = Unbundle(w52) -> (w51:dbl[], w50:dbl[])
        n5 = Bundle(w50, w51) -> (w46:cluster{dbl[], dbl[]})  [unwired: 1 in]
        n6 = call <userlib>:"dV-dI and Crit-Current.vi"("How many V sweep periods?"="How many V sweep periods?", "Input data"=w46, "dV/dI (Ic) Parameters"=w53) -> ("Ic's"=w44:T4, "dV/dI and Ic peaks"=w48:cluster{"X Subset":dbl[], "Filtered X":dbl[]}[])  [unwired: 2 in, 3 out]
        n7 = Unbundle By Name(w44) -> ("Ic (average) (A)"=w47:dbl)
        n8 = Index Array(array=w48) -> (element=w49:cluster{"X Subset":dbl[], "Filtered X":dbl[]})  [unwired: 1 in]
      }
      frame #1 {
        n9 = call <userlib>:"SC-fitting.vi"("N/SC fitting points"=w57, "Number of V-sweep periods"=w58, "Input data"=w59) -> ("Resistances"=w54:cluster{"Rn":dbl, "Rc":dbl, "Rn/Rc ratio":dbl})  [unwired: 1 in, 2 out]
        n10 = Unbundle By Name(w54) -> ("Rn"=w56:dbl, "Rc"=w55:dbl)
      }
    }
  }
  "A vs B 3" <- w30
  "dV-dI and Ic Clusters" <- w3
  "SC-fitting Clusters" <- w2
  n11 = for {
    tunnel: w30 -> [w62] mode=indexing
    tunnel: [w61] -> w26 mode=indexing
    n12 = Unbundle(w62) -> ("Filtered X"=w61:dbl[])  [unwired: 1 out]
  }
  n13 = disable-structure shown="Enabled" {
    disable-tunnel: [w63 w64] -> w18
    disable-tunnel: w17 -> [w63 w68]
    frame Disabled {
    }
    frame Enabled {
      n14 = Divide(x=w68, y="divider") -> (x/y=w66:dbl[])
      n15 = Divide(x=w66, y="divider 2") -> (x/y=w64:dbl[])
    }
  }
  n16 = Multiply(x=w17, y=w13) -> (x*y=w20:dbl[])
  n17 = disable-structure shown="Enabled" {
    disable-tunnel: w20 -> [w69 w71]
    disable-tunnel: [w69 w70] -> w19
    frame Disabled {
    }
    frame Enabled {
      n18 = Multiply(x=w71, y=2) -> (x*y=w74:dbl[])
      n19 = Divide(x=w74, y=3.141592653589793) -> (x/y=w70:dbl[])
    }
  }
  n20 = local read "Independent variable"() -> (w27:string)
  n21 = Bundle(w12, w18) -> (→"Ic":cluster{i32[], dbl[]})  [unwired: 1 in]
  n22 = Reciprocal(x=w14) -> (1/x=w8:dbl[])
  n23 = Divide(x=w8, y=w4) -> (x/y=w7:dbl[])
  n24 = Reciprocal(x=w13) -> (1/x=w5:dbl[])
  n25 = Divide(x=w5, y=w4) -> (x/y=w6:dbl[])
  n26 = Bundle(w12, w19) -> (→"IcRn":cluster{i32[], dbl[]})  [unwired: 1 in]
  n27 = Bundle(w13, w19) -> (→"IcRn vs Rn":cluster{dbl[], dbl[]})  [unwired: 1 in]
  n28 = Bundle(w13, w14) -> (→"Rc v Rn":cluster{dbl[], dbl[]})  [unwired: 1 in]
  n29 = Bundle(w12, w6) -> (w10:cluster{i32[], dbl[]})  [unwired: 1 in]
  n30 = Bundle(w12, w7) -> (w11:cluster{i32[], dbl[]})  [unwired: 1 in]
  n31 = local read "Independent variable"() -> (w21:string)
  n32 = Transpose 2D Array(2D array=w26) -> (transposed array=→"A vs B 4":dbl[][])
  n33 = property on="IcRn" class="XYGraph (strict)"("XScale.NameLbl.Text"=w21) -> ()  [unwired: 2 in, 2 out]
  n34 = property on="IcRn" class="XYGraph (strict)"("XScale.NameLbl.Text"=w21) -> ()  [unwired: 2 in, 2 out]
  n35 = Build Array(w11, w10) -> (→"Rc v Rn 2":cluster{i32[], dbl[]}[])
  n36 = property on="A vs B 3" class="XYGraph (strict)"("XScale.NameLbl.Text"=w27) -> ()  [unwired: 2 in, 2 out]
  n37 = property on="A vs B 4" class="IntGraph (strict)"("YScale.NameLbl.Text"=w27) -> ()  [unwired: 2 in, 2 out]
